vi "Test Camera + Joystick.vi"() -> ()   [LabVIEW 2019]
uses:
  Playground/Playground/Typedef/Barang.ctl
  Playground/Playground/Typedef/Kota.ctl
  <vilib>/vision/Instrument.llb/QR Code Search Options.ctl
  <vilib>/vision/Instrument.llb/Demodulation Mode.ctl
  <vilib>/vision/Instrument.llb/Cell Sample Size.ctl
  <vilib>/vision/Instrument.llb/Cell Filter Mode.ctl
  <vilib>/vision/Instrument.llb/QR Code Description Options.ctl
  <vilib>/vision/Instrument.llb/Data Matrix Polarity.ctl
  <vilib>/vision/Instrument.llb/QR Code Model Type.ctl
  <vilib>/userDefined/High Color/IMAQdx.ctl
  <vilib>/Utility/inputDevices.llb/joystickAcquire.vi
  <vilib>/Utility/inputDevices.llb/closeJoystick.vi
  <vilib>/vision/driver/NI_Vision_Acquisition_Software.lvlib
  <vilib>/vision/NI_Vision_Development_Module.lvlib
panel:
  out "axis info":T1
  out "error out":errorcluster
  in  "QR Description Options":T2={"Matrix Size (cells)"=0, "Barcode Polarity"=0, "Mirror Mode"=0, "QR Model"=3} {"Mirror Mode" items=["Auto-detect"=-2, "Normal"=0, "Mirrored"=1]; "Matrix Size (cells)" items=["Auto-detect"=0, "11x11 - Version 1 (Micro QR Only)"=11, "13x13 - Version 2 (Micro QR Only)"=13, "15x15 - Version 3 (Micro QR Only)"=15, "17x17 - Version 4 (Micro QR Only)"=17, "21x21 - Version 1"=21, "25x25 - Version 2"=25, "29x29 - Version 3"=29, "33x33 - Version 4"=33, "37x37 - Version 5"=37, "41x41 - Version 6"=41, "45x45 - Version 7"=45, "49x49 - Version 8"=49, "53x53 - Version 9"=53, "57x57 - Version 10"=57, "61x61 - Version 11"=61, "65x65 - Version 12"=65, "69x69 - Version 13"=69, "73x73 - Version 14"=73, "77x77 - Version 15"=77, "81x81 - Version 16"=81, "85x85 - Version 17"=85, "89x89 - Version 18"=89, "93x93 - Version 19"=93, "97x97 - Version 20"=97, "101x101 - Version 21"=101, "105x105 - Version 22"=105, "109x109 - Version 23"=109, "113x113 - Version 24"=113, "117x117 - Version 25"=117, "121x121 - Version 26"=121, "125x125 - Version 27"=125, "129x129 - Version 28"=129, "133x133 - Version 29"=133, "137x137 - Version 30"=137, "141x141 - Version 31"=141, "145x145 - Version 32"=145, "149x149 - Version 33"=149, "153x153 - Version 34"=153, "157x157 - Version 35"=157, "161x161 - Version 36"=161, "165x165 - Version 37"=165, "169x169 -  Version 38"=169, "173x173 - Version 39"=173, "177x177 - Version 40"=177]; "QR Model" items=["Auto-detect", "Micro", "Model 1", "Model 2"]; "Barcode Polarity" items=["Auto-detect"=-2, "Black on White"=0, "White on Black"=1]}
  in  "QR Code Cell Size (pixels)":cluster{"Minimum Size":u32, "Maximum Size":u32}={"Minimum Size"=3, "Maximum Size"=7}
  in  "QR Search Options":T5={"Rotation Mode"=enum."Unlimited", "Skip Location?"=FALSE, "Edge Threshold"=30, "Demodulation Mode"=0, "Cell Sample Size"=3, "Cell Filter Mode"=-2, "Skew Degrees Allowed"=5} {"Cell Filter Mode" items=["Auto-detect"=-2, "Average"=0, "Median"=1, "Central Average"=2, "High Average"=3, "Low Average"=4, "Very High Average"=5, "Very Low Average"=6, "All Filters"=8]; "Cell Sample Size" items=["Auto-detect"=-2, "1x1"=1, "2x2"=2, "3x3"=3, "4x4"=4, "5x5"=5, "6x6"=6, "7x7"=7]; "Demodulation Mode" items=["Auto-detect"=-2, "Histogram"=0, "Local Contrast"=1, "Combination"=2, "All"=3]}
  out "appended array":cluster{"Kota":T9, T10[], bool[]}[](array[cluster])
  out "output cluster":cluster{"Kota":T9, T10[], bool[]}
  out "Saved":bool
  out "Data num":dbl
  out "Image":T11(plugin-control)
  out "Found?":bool
  out "Data":string
  out "ROI":T11(plugin-control)
  in  "HSV Sample":T12(array[cluster])=[{"Red or Hue Range"={"Lower value"=240, "Upper value"=253}, "Green or Sat Range"={"Lower value"=4, "Upper value"=35}, "Blue or Luma or Val or Inten Range"={"Lower value"=115, "Upper value"=160}}, {"Red or Hue Range"={"Lower value"=102, "Upper value"=140}, "Green or Sat Range"={"Lower value"=6, "Upper value"=26}, "Blue or Luma or Val or Inten Range"={"Lower value"=112, "Upper value"=142}}, {"Red or Hue Range"={"Lower value"=149, "Upper value"=166}, "Green or Sat Range"={"Lower value"=6, "Upper value"=28}, "Blue or Luma or Val or Inten Range"={"Lower value"=106, "Upper value"=132}}, {"Red or Hue Range"={"Lower value"=146, "Upper value"=166}, "Green or Sat Range"={"Lower value"=7, "Upper value"=29}, "Blue or Luma or Val or Inten Range"={"Lower value"=108, "Upper value"=131}}, {"Red or Hue Range"={"Lower value"=146, "Upper value"=170}, "Green or Sat Range"={"Lower value"=7, "Upper value"=28}, "Blue or Luma or Val or Inten Range"={"Lower value"=106, "Upper value"=130}}, {"Red or Hue Range"={"Lower value"=146, "Upper value"=165}, "Green or Sat Range"={"Lower value"=6, "Upper value"=27}, "Blue or Luma or Val or Inten Range"={"Lower value"=106, "Upper value"=132}}, {"Red or Hue Range"={"Lower value"=145, "Upper value"=166}, "Green or Sat Range"={"Lower value"=6, "Upper value"=28}, "Blue or Luma or Val or Inten Range"={"Lower value"=108, "Upper value"=131}}, {"Red or Hue Range"={"Lower value"=146, "Upper value"=168}, "Green or Sat Range"={"Lower value"=7, "Upper value"=31}, "Blue or Luma or Val or Inten Range"={"Lower value"=108, "Upper value"=129}}, {"Red or Hue Range"={"Lower value"=146, "Upper value"=170}, "Green or Sat Range"={"Lower value"=7, "Upper value"=28}, "Blue or Luma or Val or Inten Range"={"Lower value"=108, "Upper value"=130}}, {"Red or Hue Range"={"Lower value"=146, "Upper value"=178}, "Green or Sat Range"={"Lower value"=5, "Upper value"=36}, "Blue or Luma or Val or Inten Range"={"Lower value"=105, "Upper value"=134}}, {"Red or Hue Range"={"Lower value"=142, "Upper value"=178}, "Green or Sat Range"={"Lower value"=4, "Upper value"=32}, "Blue or Luma or Val or Inten Range"={"Lower value"=104, "Upper value"=133}}, {"Red or Hue Range"={"Lower value"=149, "Upper value"=166}, "Green or Sat Range"={"Lower value"=10, "Upper value"=37}, "Blue or Luma or Val or Inten Range"={"Lower value"=110, "Upper value"=137}}, {"Red or Hue Range"={"Lower value"=149, "Upper value"=170}, "Green or Sat Range"={"Lower value"=9, "Upper value"=39}, "Blue or Luma or Val or Inten Range"={"Lower value"=110, "Upper value"=139}}, {"Red or Hue Range"={"Lower value"=106, "Upper value"=137}, "Green or Sat Range"={"Lower value"=7, "Upper value"=25}, "Blue or Luma or Val or Inten Range"={"Lower value"=114, "Upper value"=147}}, {"Red or Hue Range"={"Lower value"=228, "Upper value"=253}, "Green or Sat Range"={"Lower value"=4, "Upper value"=37}, "Blue or Luma or Val or Inten Range"={"Lower value"=114, "Upper value"=164}}, {"Red or Hue Range"={"Lower value"=237, "Upper value"=253}, "Green or Sat Range"={"Lower value"=6, "Upper value"=36}, "Blue or Luma or Val or Inten Range"={"Lower value"=114, "Upper value"=159}}, {"Red or Hue Range"={"Lower value"=0, "Upper value"=253}, "Green or Sat Range"={"Lower value"=6, "Upper value"=37}, "Blue or Luma or Val or Inten Range"={"Lower value"=114, "Upper value"=161}}, {"Red or Hue Range"={"Lower value"=140, "Upper value"=253}, "Green or Sat Range"={"Lower value"=2, "Upper value"=43}, "Blue or Luma or Val or Inten Range"={"Lower value"=109, "Upper value"=186}}, {"Red or Hue Range"={"Lower value"=140, "Upper value"=253}, "Green or Sat Range"={"Lower value"=2, "Upper value"=44}, "Blue or Luma or Val or Inten Range"={"Lower value"=108, "Upper value"=193}}, {"Red or Hue Range"={"Lower value"=0, "Upper value"=253}, "Green or Sat Range"={"Lower value"=2, "Upper value"=41}, "Blue or Luma or Val or Inten Range"={"Lower value"=108, "Upper value"=188}}, {"Red or Hue Range"={"Lower value"=0, "Upper value"=253}, "Green or Sat Range"={"Lower value"=2, "Upper value"=41}, "Blue or Luma or Val or Inten Range"={"Lower value"=109, "Upper value"=187}}, {"Red or Hue Range"={"Lower value"=239, "Upper value"=252}, "Green or Sat Range"={"Lower value"=14, "Upper value"=36}, "Blue or Luma or Val or Inten Range"={"Lower value"=132, "Upper value"=160}}, {"Red or Hue Range"={"Lower value"=110, "Upper value"=132}, "Green or Sat Range"={"Lower value"=7, "Upper value"=21}, "Blue or Luma or Val or Inten Range"={"Lower value"=115, "Upper value"=130}}, {"Red or Hue Range"={"Lower value"=145, "Upper value"=170}, "Green or Sat Range"={"Lower value"=10, "Upper value"=29}, "Blue or Luma or Val or Inten Range"={"Lower value"=112, "Upper value"=128}}, {"Red or Hue Range"={"Lower value"=147, "Upper value"=170}, "Green or Sat Range"={"Lower value"=8, "Upper value"=27}, "Blue or Luma or Val or Inten Range"={"Lower value"=111, "Upper value"=127}}, {"Red or Hue Range"={"Lower value"=150, "Upper value"=170}, "Green or Sat Range"={"Lower value"=10, "Upper value"=27}, "Blue or Luma or Val or Inten Range"={"Lower value"=113, "Upper value"=126}}, {"Red or Hue Range"={"Lower value"=149, "Upper value"=170}, "Green or Sat Range"={"Lower value"=8, "Upper value"=29}, "Blue or Luma or Val or Inten Range"={"Lower value"=112, "Upper value"=126}}, {"Red or Hue Range"={"Lower value"=109, "Upper value"=131}, "Green or Sat Range"={"Lower value"=7, "Upper value"=21}, "Blue or Luma or Val or Inten Range"={"Lower value"=115, "Upper value"=131}}, {"Red or Hue Range"={"Lower value"=109, "Upper value"=132}, "Green or Sat Range"={"Lower value"=7, "Upper value"=21}, "Blue or Luma or Val or Inten Range"={"Lower value"=115, "Upper value"=130}}, {"Red or Hue Range"={"Lower value"=109, "Upper value"=131}, "Green or Sat Range"={"Lower value"=8, "Upper value"=21}, "Blue or Luma or Val or Inten Range"={"Lower value"=115, "Upper value"=130}}, {"Red or Hue Range"={"Lower value"=239, "Upper value"=253}, "Green or Sat Range"={"Lower value"=15, "Upper value"=37}, "Blue or Luma or Val or Inten Range"={"Lower value"=129, "Upper value"=163}}, {"Red or Hue Range"={"Lower value"=239, "Upper value"=251}, "Green or Sat Range"={"Lower value"=15, "Upper value"=38}, "Blue or Luma or Val or Inten Range"={"Lower value"=128, "Upper value"=163}}, {"Red or Hue Range"={"Lower value"=239, "Upper value"=252}, "Green or Sat Range"={"Lower value"=15, "Upper value"=37}, "Blue or Luma or Val or Inten Range"={"Lower value"=128, "Upper value"=164}}, {"Red or Hue Range"={"Lower value"=240, "Upper value"=252}, "Green or Sat Range"={"Lower value"=17, "Upper value"=37}, "Blue or Luma or Val or Inten Range"={"Lower value"=132, "Upper value"=163}}, {"Red or Hue Range"={"Lower value"=239, "Upper value"=251}, "Green or Sat Range"={"Lower value"=16, "Upper value"=38}, "Blue or Luma or Val or Inten Range"={"Lower value"=132, "Upper value"=164}}, {"Red or Hue Range"={"Lower value"=239, "Upper value"=253}, "Green or Sat Range"={"Lower value"=16, "Upper value"=37}, "Blue or Luma or Val or Inten Range"={"Lower value"=134, "Upper value"=165}}, {"Red or Hue Range"={"Lower value"=245, "Upper value"=251}, "Green or Sat Range"={"Lower value"=59, "Upper value"=85}, "Blue or Luma or Val or Inten Range"={"Lower value"=171, "Upper value"=194}}, {"Red or Hue Range"={"Lower value"=112, "Upper value"=124}, "Green or Sat Range"={"Lower value"=23, "Upper value"=37}, "Blue or Luma or Val or Inten Range"={"Lower value"=121, "Upper value"=145}}, {"Red or Hue Range"={"Lower value"=112, "Upper value"=126}, "Green or Sat Range"={"Lower value"=23, "Upper value"=37}, "Blue or Luma or Val or Inten Range"={"Lower value"=121, "Upper value"=143}}, {"Red or Hue Range"={"Lower value"=112, "Upper value"=126}, "Green or Sat Range"={"Lower value"=23, "Upper value"=39}, "Blue or Luma or Val or Inten Range"={"Lower value"=119, "Upper value"=144}}, {"Red or Hue Range"={"Lower value"=112, "Upper value"=126}, "Green or Sat Range"={"Lower value"=24, "Upper value"=37}, "Blue or Luma or Val or Inten Range"={"Lower value"=118, "Upper value"=144}}, {"Red or Hue Range"={"Lower value"=245, "Upper value"=251}, "Green or Sat Range"={"Lower value"=63, "Upper value"=83}, "Blue or Luma or Val or Inten Range"={"Lower value"=173, "Upper value"=192}}, {"Red or Hue Range"={"Lower value"=245, "Upper value"=251}, "Green or Sat Range"={"Lower value"=60, "Upper value"=85}, "Blue or Luma or Val or Inten Range"={"Lower value"=172, "Upper value"=194}}, {"Red or Hue Range"={"Lower value"=245, "Upper value"=251}, "Green or Sat Range"={"Lower value"=57, "Upper value"=81}, "Blue or Luma or Val or Inten Range"={"Lower value"=169, "Upper value"=191}}, {"Red or Hue Range"={"Lower value"=245, "Upper value"=251}, "Green or Sat Range"={"Lower value"=57, "Upper value"=88}, "Blue or Luma or Val or Inten Range"={"Lower value"=169, "Upper value"=195}}, {"Red or Hue Range"={"Lower value"=245, "Upper value"=251}, "Green or Sat Range"={"Lower value"=56, "Upper value"=83}, "Blue or Luma or Val or Inten Range"={"Lower value"=169, "Upper value"=192}}, {"Red or Hue Range"={"Lower value"=245, "Upper value"=251}, "Green or Sat Range"={"Lower value"=60, "Upper value"=87}, "Blue or Luma or Val or Inten Range"={"Lower value"=171, "Upper value"=193}}, {"Red or Hue Range"={"Lower value"=245, "Upper value"=250}, "Green or Sat Range"={"Lower value"=59, "Upper value"=86}, "Blue or Luma or Val or Inten Range"={"Lower value"=172, "Upper value"=194}}, {"Red or Hue Range"={"Lower value"=246, "Upper value"=251}, "Green or Sat Range"={"Lower value"=60, "Upper value"=87}, "Blue or Luma or Val or Inten Range"={"Lower value"=171, "Upper value"=194}}, {"Red or Hue Range"={"Lower value"=244, "Upper value"=251}, "Green or Sat Range"={"Lower value"=61, "Upper value"=87}, "Blue or Luma or Val or Inten Range"={"Lower value"=171, "Upper value"=194}}, {"Red or Hue Range"={"Lower value"=244, "Upper value"=251}, "Green or Sat Range"={"Lower value"=60, "Upper value"=87}, "Blue or Luma or Val or Inten Range"={"Lower value"=170, "Upper value"=194}}, {"Red or Hue Range"={"Lower value"=246, "Upper value"=251}, "Green or Sat Range"={"Lower value"=63, "Upper value"=86}, "Blue or Luma or Val or Inten Range"={"Lower value"=173, "Upper value"=193}}, {"Red or Hue Range"={"Lower value"=246, "Upper value"=250}, "Green or Sat Range"={"Lower value"=60, "Upper value"=87}, "Blue or Luma or Val or Inten Range"={"Lower value"=170, "Upper value"=194}}, {"Red or Hue Range"={"Lower value"=250, "Upper value"=255}, "Green or Sat Range"={"Lower value"=70, "Upper value"=125}, "Blue or Luma or Val or Inten Range"={"Lower value"=167, "Upper value"=207}}, {"Red or Hue Range"={"Lower value"=0, "Upper value"=255}, "Green or Sat Range"={"Lower value"=65, "Upper value"=121}, "Blue or Luma or Val or Inten Range"={"Lower value"=162, "Upper value"=206}}, {"Red or Hue Range"={"Lower value"=0, "Upper value"=255}, "Green or Sat Range"={"Lower value"=52, "Upper value"=164}, "Blue or Luma or Val or Inten Range"={"Lower value"=152, "Upper value"=228}}, {"Red or Hue Range"={"Lower value"=0, "Upper value"=255}, "Green or Sat Range"={"Lower value"=51, "Upper value"=166}, "Blue or Luma or Val or Inten Range"={"Lower value"=153, "Upper value"=228}}, {"Red or Hue Range"={"Lower value"=0, "Upper value"=255}, "Green or Sat Range"={"Lower value"=51, "Upper value"=172}, "Blue or Luma or Val or Inten Range"={"Lower value"=149, "Upper value"=231}}, {"Red or Hue Range"={"Lower value"=251, "Upper value"=254}, "Green or Sat Range"={"Lower value"=62, "Upper value"=110}, "Blue or Luma or Val or Inten Range"={"Lower value"=160, "Upper value"=195}}, {"Red or Hue Range"={"Lower value"=0, "Upper value"=254}, "Green or Sat Range"={"Lower value"=65, "Upper value"=110}, "Blue or Luma or Val or Inten Range"={"Lower value"=162, "Upper value"=196}}, {"Red or Hue Range"={"Lower value"=0, "Upper value"=254}, "Green or Sat Range"={"Lower value"=63, "Upper value"=109}, "Blue or Luma or Val or Inten Range"={"Lower value"=160, "Upper value"=195}}, {"Red or Hue Range"={"Lower value"=250, "Upper value"=255}, "Green or Sat Range"={"Lower value"=87, "Upper value"=125}, "Blue or Luma or Val or Inten Range"={"Lower value"=182, "Upper value"=207}}, {"Red or Hue Range"={"Lower value"=0, "Upper value"=255}, "Green or Sat Range"={"Lower value"=84, "Upper value"=127}, "Blue or Luma or Val or Inten Range"={"Lower value"=181, "Upper value"=209}}, {"Red or Hue Range"={"Lower value"=0, "Upper value"=255}, "Green or Sat Range"={"Lower value"=83, "Upper value"=125}, "Blue or Luma or Val or Inten Range"={"Lower value"=180, "Upper value"=207}}, {"Red or Hue Range"={"Lower value"=0, "Upper value"=255}, "Green or Sat Range"={"Lower value"=66, "Upper value"=144}, "Blue or Luma or Val or Inten Range"={"Lower value"=167, "Upper value"=214}}, {"Red or Hue Range"={"Lower value"=104, "Upper value"=114}, "Green or Sat Range"={"Lower value"=58, "Upper value"=113}, "Blue or Luma or Val or Inten Range"={"Lower value"=146, "Upper value"=199}}, {"Red or Hue Range"={"Lower value"=105, "Upper value"=115}, "Green or Sat Range"={"Lower value"=57, "Upper value"=114}, "Blue or Luma or Val or Inten Range"={"Lower value"=143, "Upper value"=200}}, {"Red or Hue Range"={"Lower value"=103, "Upper value"=115}, "Green or Sat Range"={"Lower value"=58, "Upper value"=111}, "Blue or Luma or Val or Inten Range"={"Lower value"=142, "Upper value"=196}}, {"Red or Hue Range"={"Lower value"=0, "Upper value"=255}, "Green or Sat Range"={"Lower value"=0, "Upper value"=255}, "Blue or Luma or Val or Inten Range"={"Lower value"=98, "Upper value"=255}}, {"Red or Hue Range"={"Lower value"=0, "Upper value"=255}, "Green or Sat Range"={"Lower value"=0, "Upper value"=255}, "Blue or Luma or Val or Inten Range"={"Lower value"=98, "Upper value"=255}}, {"Red or Hue Range"={"Lower value"=0, "Upper value"=255}, "Green or Sat Range"={"Lower value"=0, "Upper value"=255}, "Blue or Luma or Val or Inten Range"={"Lower value"=96, "Upper value"=255}}, {"Red or Hue Range"={"Lower value"=105, "Upper value"=114}, "Green or Sat Range"={"Lower value"=70, "Upper value"=120}, "Blue or Luma or Val or Inten Range"={"Lower value"=162, "Upper value"=199}}, {"Red or Hue Range"={"Lower value"=105, "Upper value"=113}, "Green or Sat Range"={"Lower value"=70, "Upper value"=116}, "Blue or Luma or Val or Inten Range"={"Lower value"=162, "Upper value"=199}}, {"Red or Hue Range"={"Lower value"=106, "Upper value"=114}, "Green or Sat Range"={"Lower value"=48, "Upper value"=68}, "Blue or Luma or Val or Inten Range"={"Lower value"=143, "Upper value"=164}}, {"Red or Hue Range"={"Lower value"=103, "Upper value"=114}, "Green or Sat Range"={"Lower value"=51, "Upper value"=68}, "Blue or Luma or Val or Inten Range"={"Lower value"=143, "Upper value"=162}}, {"Red or Hue Range"={"Lower value"=105, "Upper value"=117}, "Green or Sat Range"={"Lower value"=48, "Upper value"=70}, "Blue or Luma or Val or Inten Range"={"Lower value"=142, "Upper value"=161}}, {"Red or Hue Range"={"Lower value"=247, "Upper value"=255}, "Green or Sat Range"={"Lower value"=64, "Upper value"=148}, "Blue or Luma or Val or Inten Range"={"Lower value"=167, "Upper value"=216}}, {"Red or Hue Range"={"Lower value"=0, "Upper value"=255}, "Green or Sat Range"={"Lower value"=62, "Upper value"=145}, "Blue or Luma or Val or Inten Range"={"Lower value"=165, "Upper value"=215}}, {"Red or Hue Range"={"Lower value"=249, "Upper value"=255}, "Green or Sat Range"={"Lower value"=64, "Upper value"=142}, "Blue or Luma or Val or Inten Range"={"Lower value"=167, "Upper value"=213}}, {"Red or Hue Range"={"Lower value"=249, "Upper value"=255}, "Green or Sat Range"={"Lower value"=102, "Upper value"=143}, "Blue or Luma or Val or Inten Range"={"Lower value"=194, "Upper value"=213}}, {"Red or Hue Range"={"Lower value"=250, "Upper value"=255}, "Green or Sat Range"={"Lower value"=121, "Upper value"=146}, "Blue or Luma or Val or Inten Range"={"Lower value"=201, "Upper value"=216}}, {"Red or Hue Range"={"Lower value"=0, "Upper value"=255}, "Green or Sat Range"={"Lower value"=113, "Upper value"=255}, "Blue or Luma or Val or Inten Range"={"Lower value"=208, "Upper value"=255}}, {"Red or Hue Range"={"Lower value"=0, "Upper value"=255}, "Green or Sat Range"={"Lower value"=113, "Upper value"=255}, "Blue or Luma or Val or Inten Range"={"Lower value"=208, "Upper value"=255}}, {"Red or Hue Range"={"Lower value"=0, "Upper value"=255}, "Green or Sat Range"={"Lower value"=118, "Upper value"=255}, "Blue or Luma or Val or Inten Range"={"Lower value"=210, "Upper value"=255}}, {"Red or Hue Range"={"Lower value"=0, "Upper value"=255}, "Green or Sat Range"={"Lower value"=111, "Upper value"=255}, "Blue or Luma or Val or Inten Range"={"Lower value"=206, "Upper value"=255}}, {"Red or Hue Range"={"Lower value"=0, "Upper value"=255}, "Green or Sat Range"={"Lower value"=0, "Upper value"=255}, "Blue or Luma or Val or Inten Range"={"Lower value"=101, "Upper value"=255}}, {"Red or Hue Range"={"Lower value"=0, "Upper value"=255}, "Green or Sat Range"={"Lower value"=0, "Upper value"=255}, "Blue or Luma or Val or Inten Range"={"Lower value"=100, "Upper value"=255}}, {"Red or Hue Range"={"Lower value"=0, "Upper value"=255}, "Green or Sat Range"={"Lower value"=0, "Upper value"=255}, "Blue or Luma or Val or Inten Range"={"Lower value"=99, "Upper value"=255}}, {"Red or Hue Range"={"Lower value"=0, "Upper value"=255}, "Green or Sat Range"={"Lower value"=0, "Upper value"=255}, "Blue or Luma or Val or Inten Range"={"Lower value"=98, "Upper value"=255}}, {"Red or Hue Range"={"Lower value"=0, "Upper value"=255}, "Green or Sat Range"={"Lower value"=108, "Upper value"=188}, "Blue or Luma or Val or Inten Range"={"Lower value"=195, "Upper value"=234}}, {"Red or Hue Range"={"Lower value"=0, "Upper value"=255}, "Green or Sat Range"={"Lower value"=109, "Upper value"=190}, "Blue or Luma or Val or Inten Range"={"Lower value"=195, "Upper value"=234}}, {"Red or Hue Range"={"Lower value"=0, "Upper value"=255}, "Green or Sat Range"={"Lower value"=107, "Upper value"=196}, "Blue or Luma or Val or Inten Range"={"Lower value"=195, "Upper value"=236}}, {"Red or Hue Range"={"Lower value"=0, "Upper value"=255}, "Green or Sat Range"={"Lower value"=106, "Upper value"=195}, "Blue or Luma or Val or Inten Range"={"Lower value"=195, "Upper value"=235}}, {"Red or Hue Range"={"Lower value"=0, "Upper value"=255}, "Green or Sat Range"={"Lower value"=107, "Upper value"=189}, "Blue or Luma or Val or Inten Range"={"Lower value"=195, "Upper value"=234}}, {"Red or Hue Range"={"Lower value"=0, "Upper value"=255}, "Green or Sat Range"={"Lower value"=108, "Upper value"=190}, "Blue or Luma or Val or Inten Range"={"Lower value"=195, "Upper value"=234}}, {"Red or Hue Range"={"Lower value"=0, "Upper value"=255}, "Green or Sat Range"={"Lower value"=107, "Upper value"=194}, "Blue or Luma or Val or Inten Range"={"Lower value"=195, "Upper value"=235}}, {"Red or Hue Range"={"Lower value"=0, "Upper value"=255}, "Green or Sat Range"={"Lower value"=108, "Upper value"=190}, "Blue or Luma or Val or Inten Range"={"Lower value"=195, "Upper value"=234}}, {"Red or Hue Range"={"Lower value"=0, "Upper value"=255}, "Green or Sat Range"={"Lower value"=107, "Upper value"=188}, "Blue or Luma or Val or Inten Range"={"Lower value"=195, "Upper value"=234}}, {"Red or Hue Range"={"Lower value"=0, "Upper value"=255}, "Green or Sat Range"={"Lower value"=106, "Upper value"=190}, "Blue or Luma or Val or Inten Range"={"Lower value"=193, "Upper value"=234}}, {"Red or Hue Range"={"Lower value"=0, "Upper value"=255}, "Green or Sat Range"={"Lower value"=108, "Upper value"=190}, "Blue or Luma or Val or Inten Range"={"Lower value"=195, "Upper value"=234}}, {"Red or Hue Range"={"Lower value"=0, "Upper value"=255}, "Green or Sat Range"={"Lower value"=106, "Upper value"=194}, "Blue or Luma or Val or Inten Range"={"Lower value"=193, "Upper value"=235}}, {"Red or Hue Range"={"Lower value"=0, "Upper value"=255}, "Green or Sat Range"={"Lower value"=106, "Upper value"=190}, "Blue or Luma or Val or Inten Range"={"Lower value"=195, "Upper value"=234}}, {"Red or Hue Range"={"Lower value"=0, "Upper value"=255}, "Green or Sat Range"={"Lower value"=105, "Upper value"=187}, "Blue or Luma or Val or Inten Range"={"Lower value"=193, "Upper value"=233}}, {"Red or Hue Range"={"Lower value"=0, "Upper value"=255}, "Green or Sat Range"={"Lower value"=107, "Upper value"=189}, "Blue or Luma or Val or Inten Range"={"Lower value"=195, "Upper value"=234}}, {"Red or Hue Range"={"Lower value"=0, "Upper value"=255}, "Green or Sat Range"={"Lower value"=107, "Upper value"=190}, "Blue or Luma or Val or Inten Range"={"Lower value"=193, "Upper value"=234}}, {"Red or Hue Range"={"Lower value"=0, "Upper value"=255}, "Green or Sat Range"={"Lower value"=106, "Upper value"=185}, "Blue or Luma or Val or Inten Range"={"Lower value"=195, "Upper value"=232}}, {"Red or Hue Range"={"Lower value"=0, "Upper value"=255}, "Green or Sat Range"={"Lower value"=109, "Upper value"=186}, "Blue or Luma or Val or Inten Range"={"Lower value"=196, "Upper value"=232}}, {"Red or Hue Range"={"Lower value"=0, "Upper value"=255}, "Green or Sat Range"={"Lower value"=108, "Upper value"=187}, "Blue or Luma or Val or Inten Range"={"Lower value"=195, "Upper value"=232}}, {"Red or Hue Range"={"Lower value"=0, "Upper value"=255}, "Green or Sat Range"={"Lower value"=105, "Upper value"=184}, "Blue or Luma or Val or Inten Range"={"Lower value"=196, "Upper value"=232}}, {"Red or Hue Range"={"Lower value"=0, "Upper value"=255}, "Green or Sat Range"={"Lower value"=102, "Upper value"=189}, "Blue or Luma or Val or Inten Range"={"Lower value"=196, "Upper value"=233}}, {"Red or Hue Range"={"Lower value"=0, "Upper value"=255}, "Green or Sat Range"={"Lower value"=108, "Upper value"=185}, "Blue or Luma or Val or Inten Range"={"Lower value"=194, "Upper value"=232}}, {"Red or Hue Range"={"Lower value"=0, "Upper value"=255}, "Green or Sat Range"={"Lower value"=107, "Upper value"=186}, "Blue or Luma or Val or Inten Range"={"Lower value"=196, "Upper value"=232}}, {"Red or Hue Range"={"Lower value"=0, "Upper value"=255}, "Green or Sat Range"={"Lower value"=108, "Upper value"=186}, "Blue or Luma or Val or Inten Range"={"Lower value"=195, "Upper value"=232}}, {"Red or Hue Range"={"Lower value"=0, "Upper value"=255}, "Green or Sat Range"={"Lower value"=103, "Upper value"=186}, "Blue or Luma or Val or Inten Range"={"Lower value"=195, "Upper value"=232}}, {"Red or Hue Range"={"Lower value"=0, "Upper value"=255}, "Green or Sat Range"={"Lower value"=104, "Upper value"=186}, "Blue or Luma or Val or Inten Range"={"Lower value"=193, "Upper value"=232}}, {"Red or Hue Range"={"Lower value"=0, "Upper value"=255}, "Green or Sat Range"={"Lower value"=106, "Upper value"=186}, "Blue or Luma or Val or Inten Range"={"Lower value"=196, "Upper value"=232}}, {"Red or Hue Range"={"Lower value"=0, "Upper value"=255}, "Green or Sat Range"={"Lower value"=110, "Upper value"=186}, "Blue or Luma or Val or Inten Range"={"Lower value"=196, "Upper value"=232}}, {"Red or Hue Range"={"Lower value"=0, "Upper value"=255}, "Green or Sat Range"={"Lower value"=107, "Upper value"=184}, "Blue or Luma or Val or Inten Range"={"Lower value"=196, "Upper value"=232}}, {"Red or Hue Range"={"Lower value"=0, "Upper value"=255}, "Green or Sat Range"={"Lower value"=106, "Upper value"=191}, "Blue or Luma or Val or Inten Range"={"Lower value"=196, "Upper value"=234}}, {"Red or Hue Range"={"Lower value"=0, "Upper value"=255}, "Green or Sat Range"={"Lower value"=111, "Upper value"=190}, "Blue or Luma or Val or Inten Range"={"Lower value"=196, "Upper value"=234}}, {"Red or Hue Range"={"Lower value"=0, "Upper value"=255}, "Green or Sat Range"={"Lower value"=107, "Upper value"=185}, "Blue or Luma or Val or Inten Range"={"Lower value"=197, "Upper value"=232}}, {"Red or Hue Range"={"Lower value"=0, "Upper value"=255}, "Green or Sat Range"={"Lower value"=83, "Upper value"=118}, "Blue or Luma or Val or Inten Range"={"Lower value"=175, "Upper value"=198}}, {"Red or Hue Range"={"Lower value"=78, "Upper value"=100}, "Green or Sat Range"={"Lower value"=15, "Upper value"=36}, "Blue or Luma or Val or Inten Range"={"Lower value"=81, "Upper value"=101}}, {"Red or Hue Range"={"Lower value"=83, "Upper value"=97}, "Green or Sat Range"={"Lower value"=15, "Upper value"=37}, "Blue or Luma or Val or Inten Range"={"Lower value"=83, "Upper value"=99}}, {"Red or Hue Range"={"Lower value"=80, "Upper value"=99}, "Green or Sat Range"={"Lower value"=15, "Upper value"=36}, "Blue or Luma or Val or Inten Range"={"Lower value"=81, "Upper value"=100}}, {"Red or Hue Range"={"Lower value"=80, "Upper value"=97}, "Green or Sat Range"={"Lower value"=14, "Upper value"=36}, "Blue or Luma or Val or Inten Range"={"Lower value"=81, "Upper value"=97}}, {"Red or Hue Range"={"Lower value"=83, "Upper value"=100}, "Green or Sat Range"={"Lower value"=15, "Upper value"=37}, "Blue or Luma or Val or Inten Range"={"Lower value"=83, "Upper value"=100}}, {"Red or Hue Range"={"Lower value"=81, "Upper value"=99}, "Green or Sat Range"={"Lower value"=15, "Upper value"=34}, "Blue or Luma or Val or Inten Range"={"Lower value"=82, "Upper value"=101}}, {"Red or Hue Range"={"Lower value"=83, "Upper value"=98}, "Green or Sat Range"={"Lower value"=12, "Upper value"=36}, "Blue or Luma or Val or Inten Range"={"Lower value"=81, "Upper value"=101}}, {"Red or Hue Range"={"Lower value"=83, "Upper value"=99}, "Green or Sat Range"={"Lower value"=15, "Upper value"=41}, "Blue or Luma or Val or Inten Range"={"Lower value"=82, "Upper value"=100}}, {"Red or Hue Range"={"Lower value"=81, "Upper value"=97}, "Green or Sat Range"={"Lower value"=15, "Upper value"=37}, "Blue or Luma or Val or Inten Range"={"Lower value"=81, "Upper value"=100}}, {"Red or Hue Range"={"Lower value"=78, "Upper value"=96}, "Green or Sat Range"={"Lower value"=15, "Upper value"=37}, "Blue or Luma or Val or Inten Range"={"Lower value"=81, "Upper value"=101}}, {"Red or Hue Range"={"Lower value"=0, "Upper value"=255}, "Green or Sat Range"={"Lower value"=81, "Upper value"=119}, "Blue or Luma or Val or Inten Range"={"Lower value"=173, "Upper value"=200}}, {"Red or Hue Range"={"Lower value"=0, "Upper value"=255}, "Green or Sat Range"={"Lower value"=81, "Upper value"=118}, "Blue or Luma or Val or Inten Range"={"Lower value"=175, "Upper value"=198}}, {"Red or Hue Range"={"Lower value"=0, "Upper value"=255}, "Green or Sat Range"={"Lower value"=81, "Upper value"=119}, "Blue or Luma or Val or Inten Range"={"Lower value"=174, "Upper value"=201}}, {"Red or Hue Range"={"Lower value"=0, "Upper value"=255}, "Green or Sat Range"={"Lower value"=83, "Upper value"=123}, "Blue or Luma or Val or Inten Range"={"Lower value"=177, "Upper value"=201}}, {"Red or Hue Range"={"Lower value"=0, "Upper value"=255}, "Green or Sat Range"={"Lower value"=79, "Upper value"=118}, "Blue or Luma or Val or Inten Range"={"Lower value"=173, "Upper value"=198}}, {"Red or Hue Range"={"Lower value"=0, "Upper value"=255}, "Green or Sat Range"={"Lower value"=79, "Upper value"=118}, "Blue or Luma or Val or Inten Range"={"Lower value"=173, "Upper value"=199}}, {"Red or Hue Range"={"Lower value"=0, "Upper value"=255}, "Green or Sat Range"={"Lower value"=75, "Upper value"=120}, "Blue or Luma or Val or Inten Range"={"Lower value"=171, "Upper value"=199}}, {"Red or Hue Range"={"Lower value"=0, "Upper value"=255}, "Green or Sat Range"={"Lower value"=84, "Upper value"=117}, "Blue or Luma or Val or Inten Range"={"Lower value"=175, "Upper value"=200}}, {"Red or Hue Range"={"Lower value"=0, "Upper value"=255}, "Green or Sat Range"={"Lower value"=82, "Upper value"=121}, "Blue or Luma or Val or Inten Range"={"Lower value"=172, "Upper value"=199}}, {"Red or Hue Range"={"Lower value"=0, "Upper value"=255}, "Green or Sat Range"={"Lower value"=10, "Upper value"=151}, "Blue or Luma or Val or Inten Range"={"Lower value"=160, "Upper value"=223}}, {"Red or Hue Range"={"Lower value"=0, "Upper value"=255}, "Green or Sat Range"={"Lower value"=16, "Upper value"=165}, "Blue or Luma or Val or Inten Range"={"Lower value"=155, "Upper value"=229}}, {"Red or Hue Range"={"Lower value"=0, "Upper value"=255}, "Green or Sat Range"={"Lower value"=25, "Upper value"=160}, "Blue or Luma or Val or Inten Range"={"Lower value"=152, "Upper value"=229}}, {"Red or Hue Range"={"Lower value"=0, "Upper value"=255}, "Green or Sat Range"={"Lower value"=10, "Upper value"=154}, "Blue or Luma or Val or Inten Range"={"Lower value"=157, "Upper value"=224}}, {"Red or Hue Range"={"Lower value"=0, "Upper value"=255}, "Green or Sat Range"={"Lower value"=22, "Upper value"=158}, "Blue or Luma or Val or Inten Range"={"Lower value"=155, "Upper value"=226}}, {"Red or Hue Range"={"Lower value"=0, "Upper value"=255}, "Green or Sat Range"={"Lower value"=26, "Upper value"=148}, "Blue or Luma or Val or Inten Range"={"Lower value"=151, "Upper value"=221}}, {"Red or Hue Range"={"Lower value"=0, "Upper value"=255}, "Green or Sat Range"={"Lower value"=14, "Upper value"=150}, "Blue or Luma or Val or Inten Range"={"Lower value"=161, "Upper value"=222}}, {"Red or Hue Range"={"Lower value"=0, "Upper value"=254}, "Green or Sat Range"={"Lower value"=46, "Upper value"=86}, "Blue or Luma or Val or Inten Range"={"Lower value"=102, "Upper value"=159}}, {"Red or Hue Range"={"Lower value"=0, "Upper value"=254}, "Green or Sat Range"={"Lower value"=45, "Upper value"=86}, "Blue or Luma or Val or Inten Range"={"Lower value"=98, "Upper value"=156}}, {"Red or Hue Range"={"Lower value"=0, "Upper value"=254}, "Green or Sat Range"={"Lower value"=35, "Upper value"=86}, "Blue or Luma or Val or Inten Range"={"Lower value"=92, "Upper value"=158}}, {"Red or Hue Range"={"Lower value"=0, "Upper value"=254}, "Green or Sat Range"={"Lower value"=45, "Upper value"=89}, "Blue or Luma or Val or Inten Range"={"Lower value"=100, "Upper value"=163}}, {"Red or Hue Range"={"Lower value"=0, "Upper value"=254}, "Green or Sat Range"={"Lower value"=42, "Upper value"=85}, "Blue or Luma or Val or Inten Range"={"Lower value"=100, "Upper value"=163}}, {"Red or Hue Range"={"Lower value"=0, "Upper value"=254}, "Green or Sat Range"={"Lower value"=46, "Upper value"=87}, "Blue or Luma or Val or Inten Range"={"Lower value"=102, "Upper value"=162}}, {"Red or Hue Range"={"Lower value"=0, "Upper value"=254}, "Green or Sat Range"={"Lower value"=47, "Upper value"=88}, "Blue or Luma or Val or Inten Range"={"Lower value"=102, "Upper value"=153}}, {"Red or Hue Range"={"Lower value"=0, "Upper value"=254}, "Green or Sat Range"={"Lower value"=46, "Upper value"=89}, "Blue or Luma or Val or Inten Range"={"Lower value"=101, "Upper value"=155}}, {"Red or Hue Range"={"Lower value"=0, "Upper value"=254}, "Green or Sat Range"={"Lower value"=41, "Upper value"=86}, "Blue or Luma or Val or Inten Range"={"Lower value"=98, "Upper value"=162}}, {"Red or Hue Range"={"Lower value"=0, "Upper value"=254}, "Green or Sat Range"={"Lower value"=46, "Upper value"=85}, "Blue or Luma or Val or Inten Range"={"Lower value"=102, "Upper value"=159}}, {"Red or Hue Range"={"Lower value"=0, "Upper value"=254}, "Green or Sat Range"={"Lower value"=47, "Upper value"=89}, "Blue or Luma or Val or Inten Range"={"Lower value"=99, "Upper value"=157}}, {"Red or Hue Range"={"Lower value"=0, "Upper value"=254}, "Green or Sat Range"={"Lower value"=42, "Upper value"=87}, "Blue or Luma or Val or Inten Range"={"Lower value"=95, "Upper value"=160}}, {"Red or Hue Range"={"Lower value"=0, "Upper value"=254}, "Green or Sat Range"={"Lower value"=46, "Upper value"=89}, "Blue or Luma or Val or Inten Range"={"Lower value"=102, "Upper value"=157}}, {"Red or Hue Range"={"Lower value"=0, "Upper value"=254}, "Green or Sat Range"={"Lower value"=43, "Upper value"=87}, "Blue or Luma or Val or Inten Range"={"Lower value"=100, "Upper value"=158}}, {"Red or Hue Range"={"Lower value"=0, "Upper value"=254}, "Green or Sat Range"={"Lower value"=41, "Upper value"=85}, "Blue or Luma or Val or Inten Range"={"Lower value"=96, "Upper value"=160}}, {"Red or Hue Range"={"Lower value"=0, "Upper value"=254}, "Green or Sat Range"={"Lower value"=37, "Upper value"=87}, "Blue or Luma or Val or Inten Range"={"Lower value"=95, "Upper value"=160}}, {"Red or Hue Range"={"Lower value"=0, "Upper value"=254}, "Green or Sat Range"={"Lower value"=41, "Upper value"=86}, "Blue or Luma or Val or Inten Range"={"Lower value"=98, "Upper value"=158}}, {"Red or Hue Range"={"Lower value"=0, "Upper value"=255}, "Green or Sat Range"={"Lower value"=51, "Upper value"=210}, "Blue or Luma or Val or Inten Range"={"Lower value"=162, "Upper value"=241}}, {"Red or Hue Range"={"Lower value"=86, "Upper value"=121}, "Green or Sat Range"={"Lower value"=45, "Upper value"=137}, "Blue or Luma or Val or Inten Range"={"Lower value"=151, "Upper value"=201}}, {"Red or Hue Range"={"Lower value"=85, "Upper value"=120}, "Green or Sat Range"={"Lower value"=55, "Upper value"=135}, "Blue or Luma or Val or Inten Range"={"Lower value"=154, "Upper value"=200}}, {"Red or Hue Range"={"Lower value"=85, "Upper value"=120}, "Green or Sat Range"={"Lower value"=57, "Upper value"=135}, "Blue or Luma or Val or Inten Range"={"Lower value"=153, "Upper value"=199}}, {"Red or Hue Range"={"Lower value"=85, "Upper value"=122}, "Green or Sat Range"={"Lower value"=45, "Upper value"=136}, "Blue or Luma or Val or Inten Range"={"Lower value"=150, "Upper value"=201}}, {"Red or Hue Range"={"Lower value"=85, "Upper value"=121}, "Green or Sat Range"={"Lower value"=57, "Upper value"=137}, "Blue or Luma or Val or Inten Range"={"Lower value"=151, "Upper value"=200}}, {"Red or Hue Range"={"Lower value"=83, "Upper value"=120}, "Green or Sat Range"={"Lower value"=45, "Upper value"=134}, "Blue or Luma or Val or Inten Range"={"Lower value"=150, "Upper value"=204}}, {"Red or Hue Range"={"Lower value"=86, "Upper value"=119}, "Green or Sat Range"={"Lower value"=51, "Upper value"=138}, "Blue or Luma or Val or Inten Range"={"Lower value"=152, "Upper value"=201}}, {"Red or Hue Range"={"Lower value"=85, "Upper value"=121}, "Green or Sat Range"={"Lower value"=45, "Upper value"=136}, "Blue or Luma or Val or Inten Range"={"Lower value"=151, "Upper value"=202}}, {"Red or Hue Range"={"Lower value"=84, "Upper value"=118}, "Green or Sat Range"={"Lower value"=35, "Upper value"=136}, "Blue or Luma or Val or Inten Range"={"Lower value"=148, "Upper value"=204}}, {"Red or Hue Range"={"Lower value"=85, "Upper value"=121}, "Green or Sat Range"={"Lower value"=45, "Upper value"=136}, "Blue or Luma or Val or Inten Range"={"Lower value"=151, "Upper value"=200}}, {"Red or Hue Range"={"Lower value"=82, "Upper value"=126}, "Green or Sat Range"={"Lower value"=21, "Upper value"=155}, "Blue or Luma or Val or Inten Range"={"Lower value"=142, "Upper value"=230}}, {"Red or Hue Range"={"Lower value"=85, "Upper value"=127}, "Green or Sat Range"={"Lower value"=21, "Upper value"=151}, "Blue or Luma or Val or Inten Range"={"Lower value"=144, "Upper value"=228}}, {"Red or Hue Range"={"Lower value"=81, "Upper value"=127}, "Green or Sat Range"={"Lower value"=17, "Upper value"=145}, "Blue or Luma or Val or Inten Range"={"Lower value"=142, "Upper value"=227}}, {"Red or Hue Range"={"Lower value"=85, "Upper value"=127}, "Green or Sat Range"={"Lower value"=25, "Upper value"=142}, "Blue or Luma or Val or Inten Range"={"Lower value"=147, "Upper value"=226}}, {"Red or Hue Range"={"Lower value"=80, "Upper value"=129}, "Green or Sat Range"={"Lower value"=23, "Upper value"=151}, "Blue or Luma or Val or Inten Range"={"Lower value"=147, "Upper value"=229}}, {"Red or Hue Range"={"Lower value"=75, "Upper value"=126}, "Green or Sat Range"={"Lower value"=23, "Upper value"=152}, "Blue or Luma or Val or Inten Range"={"Lower value"=144, "Upper value"=228}}, {"Red or Hue Range"={"Lower value"=85, "Upper value"=127}, "Green or Sat Range"={"Lower value"=21, "Upper value"=145}, "Blue or Luma or Val or Inten Range"={"Lower value"=139, "Upper value"=226}}, {"Red or Hue Range"={"Lower value"=85, "Upper value"=127}, "Green or Sat Range"={"Lower value"=20, "Upper value"=147}, "Blue or Luma or Val or Inten Range"={"Lower value"=149, "Upper value"=229}}, {"Red or Hue Range"={"Lower value"=85, "Upper value"=127}, "Green or Sat Range"={"Lower value"=21, "Upper value"=151}, "Blue or Luma or Val or Inten Range"={"Lower value"=144, "Upper value"=227}}, {"Red or Hue Range"={"Lower value"=85, "Upper value"=127}, "Green or Sat Range"={"Lower value"=22, "Upper value"=149}, "Blue or Luma or Val or Inten Range"={"Lower value"=145, "Upper value"=226}}, {"Red or Hue Range"={"Lower value"=85, "Upper value"=129}, "Green or Sat Range"={"Lower value"=21, "Upper value"=141}, "Blue or Luma or Val or Inten Range"={"Lower value"=146, "Upper value"=227}}, {"Red or Hue Range"={"Lower value"=85, "Upper value"=127}, "Green or Sat Range"={"Lower value"=23, "Upper value"=146}, "Blue or Luma or Val or Inten Range"={"Lower value"=148, "Upper value"=228}}, {"Red or Hue Range"={"Lower value"=83, "Upper value"=130}, "Green or Sat Range"={"Lower value"=29, "Upper value"=150}, "Blue or Luma or Val or Inten Range"={"Lower value"=146, "Upper value"=227}}, {"Red or Hue Range"={"Lower value"=85, "Upper value"=127}, "Green or Sat Range"={"Lower value"=23, "Upper value"=142}, "Blue or Luma or Val or Inten Range"={"Lower value"=145, "Upper value"=226}}, {"Red or Hue Range"={"Lower value"=83, "Upper value"=128}, "Green or Sat Range"={"Lower value"=21, "Upper value"=150}, "Blue or Luma or Val or Inten Range"={"Lower value"=147, "Upper value"=225}}, {"Red or Hue Range"={"Lower value"=0, "Upper value"=255}, "Green or Sat Range"={"Lower value"=55, "Upper value"=207}, "Blue or Luma or Val or Inten Range"={"Lower value"=163, "Upper value"=239}}, {"Red or Hue Range"={"Lower value"=0, "Upper value"=255}, "Green or Sat Range"={"Lower value"=50, "Upper value"=203}, "Blue or Luma or Val or Inten Range"={"Lower value"=159, "Upper value"=238}}, {"Red or Hue Range"={"Lower value"=0, "Upper value"=255}, "Green or Sat Range"={"Lower value"=47, "Upper value"=207}, "Blue or Luma or Val or Inten Range"={"Lower value"=162, "Upper value"=240}}, {"Red or Hue Range"={"Lower value"=0, "Upper value"=255}, "Green or Sat Range"={"Lower value"=53, "Upper value"=205}, "Blue or Luma or Val or Inten Range"={"Lower value"=160, "Upper value"=239}}, {"Red or Hue Range"={"Lower value"=0, "Upper value"=255}, "Green or Sat Range"={"Lower value"=47, "Upper value"=212}, "Blue or Luma or Val or Inten Range"={"Lower value"=160, "Upper value"=242}}, {"Red or Hue Range"={"Lower value"=0, "Upper value"=255}, "Green or Sat Range"={"Lower value"=47, "Upper value"=202}, "Blue or Luma or Val or Inten Range"={"Lower value"=160, "Upper value"=238}}, {"Red or Hue Range"={"Lower value"=0, "Upper value"=255}, "Green or Sat Range"={"Lower value"=47, "Upper value"=207}, "Blue or Luma or Val or Inten Range"={"Lower value"=161, "Upper value"=239}}, {"Red or Hue Range"={"Lower value"=0, "Upper value"=255}, "Green or Sat Range"={"Lower value"=52, "Upper value"=224}, "Blue or Luma or Val or Inten Range"={"Lower value"=163, "Upper value"=246}}, {"Red or Hue Range"={"Lower value"=0, "Upper value"=255}, "Green or Sat Range"={"Lower value"=48, "Upper value"=224}, "Blue or Luma or Val or Inten Range"={"Lower value"=156, "Upper value"=246}}, {"Red or Hue Range"={"Lower value"=0, "Upper value"=255}, "Green or Sat Range"={"Lower value"=54, "Upper value"=207}, "Blue or Luma or Val or Inten Range"={"Lower value"=163, "Upper value"=240}}, {"Red or Hue Range"={"Lower value"=0, "Upper value"=255}, "Green or Sat Range"={"Lower value"=57, "Upper value"=212}, "Blue or Luma or Val or Inten Range"={"Lower value"=162, "Upper value"=241}}, {"Red or Hue Range"={"Lower value"=0, "Upper value"=255}, "Green or Sat Range"={"Lower value"=50, "Upper value"=225}, "Blue or Luma or Val or Inten Range"={"Lower value"=164, "Upper value"=246}}, {"Red or Hue Range"={"Lower value"=0, "Upper value"=255}, "Green or Sat Range"={"Lower value"=48, "Upper value"=208}, "Blue or Luma or Val or Inten Range"={"Lower value"=157, "Upper value"=240}}, {"Red or Hue Range"={"Lower value"=0, "Upper value"=255}, "Green or Sat Range"={"Lower value"=48, "Upper value"=199}, "Blue or Luma or Val or Inten Range"={"Lower value"=165, "Upper value"=236}}, {"Red or Hue Range"={"Lower value"=0, "Upper value"=255}, "Green or Sat Range"={"Lower value"=53, "Upper value"=207}, "Blue or Luma or Val or Inten Range"={"Lower value"=161, "Upper value"=239}}, {"Red or Hue Range"={"Lower value"=0, "Upper value"=255}, "Green or Sat Range"={"Lower value"=53, "Upper value"=215}, "Blue or Luma or Val or Inten Range"={"Lower value"=155, "Upper value"=242}}, {"Red or Hue Range"={"Lower value"=0, "Upper value"=255}, "Green or Sat Range"={"Lower value"=47, "Upper value"=210}, "Blue or Luma or Val or Inten Range"={"Lower value"=164, "Upper value"=241}}, {"Red or Hue Range"={"Lower value"=0, "Upper value"=255}, "Green or Sat Range"={"Lower value"=0, "Upper value"=255}, "Blue or Luma or Val or Inten Range"={"Lower value"=60, "Upper value"=255}}, {"Red or Hue Range"={"Lower value"=0, "Upper value"=255}, "Green or Sat Range"={"Lower value"=0, "Upper value"=255}, "Blue or Luma or Val or Inten Range"={"Lower value"=60, "Upper value"=255}}, {"Red or Hue Range"={"Lower value"=0, "Upper value"=255}, "Green or Sat Range"={"Lower value"=0, "Upper value"=255}, "Blue or Luma or Val or Inten Range"={"Lower value"=61, "Upper value"=255}}, {"Red or Hue Range"={"Lower value"=0, "Upper value"=255}, "Green or Sat Range"={"Lower value"=0, "Upper value"=255}, "Blue or Luma or Val or Inten Range"={"Lower value"=60, "Upper value"=255}}, {"Red or Hue Range"={"Lower value"=0, "Upper value"=255}, "Green or Sat Range"={"Lower value"=0, "Upper value"=255}, "Blue or Luma or Val or Inten Range"={"Lower value"=110, "Upper value"=255}}, {"Red or Hue Range"={"Lower value"=0, "Upper value"=255}, "Green or Sat Range"={"Lower value"=0, "Upper value"=255}, "Blue or Luma or Val or Inten Range"={"Lower value"=108, "Upper value"=255}}, {"Red or Hue Range"={"Lower value"=0, "Upper value"=255}, "Green or Sat Range"={"Lower value"=0, "Upper value"=255}, "Blue or Luma or Val or Inten Range"={"Lower value"=108, "Upper value"=255}}, {"Red or Hue Range"={"Lower value"=0, "Upper value"=255}, "Green or Sat Range"={"Lower value"=0, "Upper value"=255}, "Blue or Luma or Val or Inten Range"={"Lower value"=106, "Upper value"=255}}, {"Red or Hue Range"={"Lower value"=0, "Upper value"=255}, "Green or Sat Range"={"Lower value"=0, "Upper value"=255}, "Blue or Luma or Val or Inten Range"={"Lower value"=108, "Upper value"=255}}, {"Red or Hue Range"={"Lower value"=0, "Upper value"=255}, "Green or Sat Range"={"Lower value"=0, "Upper value"=255}, "Blue or Luma or Val or Inten Range"={"Lower value"=107, "Upper value"=255}}, {"Red or Hue Range"={"Lower value"=0, "Upper value"=255}, "Green or Sat Range"={"Lower value"=0, "Upper value"=255}, "Blue or Luma or Val or Inten Range"={"Lower value"=106, "Upper value"=255}}, {"Red or Hue Range"={"Lower value"=0, "Upper value"=255}, "Green or Sat Range"={"Lower value"=0, "Upper value"=255}, "Blue or Luma or Val or Inten Range"={"Lower value"=109, "Upper value"=255}}, {"Red or Hue Range"={"Lower value"=0, "Upper value"=255}, "Green or Sat Range"={"Lower value"=0, "Upper value"=255}, "Blue or Luma or Val or Inten Range"={"Lower value"=109, "Upper value"=255}}, {"Red or Hue Range"={"Lower value"=0, "Upper value"=255}, "Green or Sat Range"={"Lower value"=0, "Upper value"=255}, "Blue or Luma or Val or Inten Range"={"Lower value"=109, "Upper value"=255}}, {"Red or Hue Range"={"Lower value"=0, "Upper value"=255}, "Green or Sat Range"={"Lower value"=0, "Upper value"=255}, "Blue or Luma or Val or Inten Range"={"Lower value"=109, "Upper value"=255}}, {"Red or Hue Range"={"Lower value"=0, "Upper value"=255}, "Green or Sat Range"={"Lower value"=0, "Upper value"=255}, "Blue or Luma or Val or Inten Range"={"Lower value"=106, "Upper value"=255}}, {"Red or Hue Range"={"Lower value"=0, "Upper value"=255}, "Green or Sat Range"={"Lower value"=0, "Upper value"=255}, "Blue or Luma or Val or Inten Range"={"Lower value"=108, "Upper value"=255}}, {"Red or Hue Range"={"Lower value"=0, "Upper value"=255}, "Green or Sat Range"={"Lower value"=0, "Upper value"=255}, "Blue or Luma or Val or Inten Range"={"Lower value"=110, "Upper value"=255}}, {"Red or Hue Range"={"Lower value"=0, "Upper value"=255}, "Green or Sat Range"={"Lower value"=238, "Upper value"=255}, "Blue or Luma or Val or Inten Range"={"Lower value"=249, "Upper value"=255}}, {"Red or Hue Range"={"Lower value"=0, "Upper value"=255}, "Green or Sat Range"={"Lower value"=244, "Upper value"=255}, "Blue or Luma or Val or Inten Range"={"Lower value"=251, "Upper value"=255}}, {"Red or Hue Range"={"Lower value"=0, "Upper value"=255}, "Green or Sat Range"={"Lower value"=226, "Upper value"=255}, "Blue or Luma or Val or Inten Range"={"Lower value"=245, "Upper value"=255}}, {"Red or Hue Range"={"Lower value"=0, "Upper value"=255}, "Green or Sat Range"={"Lower value"=240, "Upper value"=255}, "Blue or Luma or Val or Inten Range"={"Lower value"=250, "Upper value"=255}}, {"Red or Hue Range"={"Lower value"=0, "Upper value"=255}, "Green or Sat Range"={"Lower value"=234, "Upper value"=255}, "Blue or Luma or Val or Inten Range"={"Lower value"=248, "Upper value"=255}}, {"Red or Hue Range"={"Lower value"=0, "Upper value"=255}, "Green or Sat Range"={"Lower value"=229, "Upper value"=255}, "Blue or Luma or Val or Inten Range"={"Lower value"=246, "Upper value"=255}}, {"Red or Hue Range"={"Lower value"=0, "Upper value"=255}, "Green or Sat Range"={"Lower value"=228, "Upper value"=255}, "Blue or Luma or Val or Inten Range"={"Lower value"=246, "Upper value"=255}}, {"Red or Hue Range"={"Lower value"=0, "Upper value"=255}, "Green or Sat Range"={"Lower value"=233, "Upper value"=255}, "Blue or Luma or Val or Inten Range"={"Lower value"=246, "Upper value"=255}}, {"Red or Hue Range"={"Lower value"=0, "Upper value"=255}, "Green or Sat Range"={"Lower value"=233, "Upper value"=255}, "Blue or Luma or Val or Inten Range"={"Lower value"=247, "Upper value"=255}}, {"Red or Hue Range"={"Lower value"=0, "Upper value"=255}, "Green or Sat Range"={"Lower value"=240, "Upper value"=255}, "Blue or Luma or Val or Inten Range"={"Lower value"=249, "Upper value"=255}}, {"Red or Hue Range"={"Lower value"=0, "Upper value"=255}, "Green or Sat Range"={"Lower value"=233, "Upper value"=255}, "Blue or Luma or Val or Inten Range"={"Lower value"=247, "Upper value"=255}}, {"Red or Hue Range"={"Lower value"=0, "Upper value"=255}, "Green or Sat Range"={"Lower value"=230, "Upper value"=255}, "Blue or Luma or Val or Inten Range"={"Lower value"=245, "Upper value"=255}}, {"Red or Hue Range"={"Lower value"=0, "Upper value"=255}, "Green or Sat Range"={"Lower value"=225, "Upper value"=255}, "Blue or Luma or Val or Inten Range"={"Lower value"=243, "Upper value"=255}}, {"Red or Hue Range"={"Lower value"=0, "Upper value"=255}, "Green or Sat Range"={"Lower value"=233, "Upper value"=255}, "Blue or Luma or Val or Inten Range"={"Lower value"=247, "Upper value"=255}}, {"Red or Hue Range"={"Lower value"=0, "Upper value"=255}, "Green or Sat Range"={"Lower value"=231, "Upper value"=255}, "Blue or Luma or Val or Inten Range"={"Lower value"=247, "Upper value"=255}}, {"Red or Hue Range"={"Lower value"=0, "Upper value"=255}, "Green or Sat Range"={"Lower value"=225, "Upper value"=255}, "Blue or Luma or Val or Inten Range"={"Lower value"=243, "Upper value"=255}}, {"Red or Hue Range"={"Lower value"=0, "Upper value"=255}, "Green or Sat Range"={"Lower value"=227, "Upper value"=255}, "Blue or Luma or Val or Inten Range"={"Lower value"=244, "Upper value"=255}}, {"Red or Hue Range"={"Lower value"=0, "Upper value"=255}, "Green or Sat Range"={"Lower value"=225, "Upper value"=255}, "Blue or Luma or Val or Inten Range"={"Lower value"=244, "Upper value"=255}}, {"Red or Hue Range"={"Lower value"=0, "Upper value"=255}, "Green or Sat Range"={"Lower value"=222, "Upper value"=255}, "Blue or Luma or Val or Inten Range"={"Lower value"=244, "Upper value"=255}}, {"Red or Hue Range"={"Lower value"=0, "Upper value"=255}, "Green or Sat Range"={"Lower value"=235, "Upper value"=255}, "Blue or Luma or Val or Inten Range"={"Lower value"=247, "Upper value"=255}}, {"Red or Hue Range"={"Lower value"=0, "Upper value"=255}, "Green or Sat Range"={"Lower value"=223, "Upper value"=255}, "Blue or Luma or Val or Inten Range"={"Lower value"=243, "Upper value"=255}}, {"Red or Hue Range"={"Lower value"=0, "Upper value"=255}, "Green or Sat Range"={"Lower value"=212, "Upper value"=255}, "Blue or Luma or Val or Inten Range"={"Lower value"=237, "Upper value"=255}}, {"Red or Hue Range"={"Lower value"=0, "Upper value"=255}, "Green or Sat Range"={"Lower value"=205, "Upper value"=255}, "Blue or Luma or Val or Inten Range"={"Lower value"=234, "Upper value"=255}}, {"Red or Hue Range"={"Lower value"=0, "Upper value"=255}, "Green or Sat Range"={"Lower value"=211, "Upper value"=255}, "Blue or Luma or Val or Inten Range"={"Lower value"=235, "Upper value"=255}}, {"Red or Hue Range"={"Lower value"=0, "Upper value"=255}, "Green or Sat Range"={"Lower value"=211, "Upper value"=255}, "Blue or Luma or Val or Inten Range"={"Lower value"=236, "Upper value"=255}}, {"Red or Hue Range"={"Lower value"=0, "Upper value"=255}, "Green or Sat Range"={"Lower value"=212, "Upper value"=255}, "Blue or Luma or Val or Inten Range"={"Lower value"=237, "Upper value"=255}}, {"Red or Hue Range"={"Lower value"=0, "Upper value"=255}, "Green or Sat Range"={"Lower value"=206, "Upper value"=255}, "Blue or Luma or Val or Inten Range"={"Lower value"=234, "Upper value"=255}}, {"Red or Hue Range"={"Lower value"=0, "Upper value"=255}, "Green or Sat Range"={"Lower value"=217, "Upper value"=255}, "Blue or Luma or Val or Inten Range"={"Lower value"=239, "Upper value"=255}}, {"Red or Hue Range"={"Lower value"=0, "Upper value"=255}, "Green or Sat Range"={"Lower value"=206, "Upper value"=255}, "Blue or Luma or Val or Inten Range"={"Lower value"=234, "Upper value"=255}}, {"Red or Hue Range"={"Lower value"=0, "Upper value"=255}, "Green or Sat Range"={"Lower value"=212, "Upper value"=255}, "Blue or Luma or Val or Inten Range"={"Lower value"=237, "Upper value"=255}}, {"Red or Hue Range"={"Lower value"=0, "Upper value"=255}, "Green or Sat Range"={"Lower value"=214, "Upper value"=255}, "Blue or Luma or Val or Inten Range"={"Lower value"=238, "Upper value"=255}}, {"Red or Hue Range"={"Lower value"=0, "Upper value"=255}, "Green or Sat Range"={"Lower value"=210, "Upper value"=255}, "Blue or Luma or Val or Inten Range"={"Lower value"=236, "Upper value"=255}}, {"Red or Hue Range"={"Lower value"=0, "Upper value"=255}, "Green or Sat Range"={"Lower value"=212, "Upper value"=255}, "Blue or Luma or Val or Inten Range"={"Lower value"=237, "Upper value"=255}}, {"Red or Hue Range"={"Lower value"=0, "Upper value"=255}, "Green or Sat Range"={"Lower value"=212, "Upper value"=255}, "Blue or Luma or Val or Inten Range"={"Lower value"=237, "Upper value"=255}}, {"Red or Hue Range"={"Lower value"=0, "Upper value"=255}, "Green or Sat Range"={"Lower value"=203, "Upper value"=255}, "Blue or Luma or Val or Inten Range"={"Lower value"=233, "Upper value"=255}}, {"Red or Hue Range"={"Lower value"=0, "Upper value"=255}, "Green or Sat Range"={"Lower value"=207, "Upper value"=255}, "Blue or Luma or Val or Inten Range"={"Lower value"=228, "Upper value"=255}}, {"Red or Hue Range"={"Lower value"=0, "Upper value"=255}, "Green or Sat Range"={"Lower value"=216, "Upper value"=255}, "Blue or Luma or Val or Inten Range"={"Lower value"=239, "Upper value"=255}}, {"Red or Hue Range"={"Lower value"=0, "Upper value"=255}, "Green or Sat Range"={"Lower value"=214, "Upper value"=255}, "Blue or Luma or Val or Inten Range"={"Lower value"=238, "Upper value"=255}}, {"Red or Hue Range"={"Lower value"=0, "Upper value"=255}, "Green or Sat Range"={"Lower value"=206, "Upper value"=255}, "Blue or Luma or Val or Inten Range"={"Lower value"=234, "Upper value"=255}}, {"Red or Hue Range"={"Lower value"=0, "Upper value"=255}, "Green or Sat Range"={"Lower value"=211, "Upper value"=255}, "Blue or Luma or Val or Inten Range"={"Lower value"=237, "Upper value"=255}}, {"Red or Hue Range"={"Lower value"=0, "Upper value"=255}, "Green or Sat Range"={"Lower value"=207, "Upper value"=255}, "Blue or Luma or Val or Inten Range"={"Lower value"=231, "Upper value"=255}}, {"Red or Hue Range"={"Lower value"=0, "Upper value"=255}, "Green or Sat Range"={"Lower value"=212, "Upper value"=255}, "Blue or Luma or Val or Inten Range"={"Lower value"=237, "Upper value"=255}}, {"Red or Hue Range"={"Lower value"=0, "Upper value"=255}, "Green or Sat Range"={"Lower value"=210, "Upper value"=255}, "Blue or Luma or Val or Inten Range"={"Lower value"=236, "Upper value"=255}}, {"Red or Hue Range"={"Lower value"=0, "Upper value"=255}, "Green or Sat Range"={"Lower value"=214, "Upper value"=255}, "Blue or Luma or Val or Inten Range"={"Lower value"=238, "Upper value"=255}}, {"Red or Hue Range"={"Lower value"=0, "Upper value"=255}, "Green or Sat Range"={"Lower value"=212, "Upper value"=255}, "Blue or Luma or Val or Inten Range"={"Lower value"=236, "Upper value"=255}}, {"Red or Hue Range"={"Lower value"=0, "Upper value"=255}, "Green or Sat Range"={"Lower value"=205, "Upper value"=255}, "Blue or Luma or Val or Inten Range"={"Lower value"=234, "Upper value"=255}}, {"Red or Hue Range"={"Lower value"=0, "Upper value"=255}, "Green or Sat Range"={"Lower value"=53, "Upper value"=255}, "Blue or Luma or Val or Inten Range"={"Lower value"=163, "Upper value"=255}}, {"Red or Hue Range"={"Lower value"=0, "Upper value"=255}, "Green or Sat Range"={"Lower value"=47, "Upper value"=255}, "Blue or Luma or Val or Inten Range"={"Lower value"=163, "Upper value"=255}}, {"Red or Hue Range"={"Lower value"=0, "Upper value"=255}, "Green or Sat Range"={"Lower value"=57, "Upper value"=255}, "Blue or Luma or Val or Inten Range"={"Lower value"=163, "Upper value"=255}}, {"Red or Hue Range"={"Lower value"=0, "Upper value"=255}, "Green or Sat Range"={"Lower value"=51, "Upper value"=255}, "Blue or Luma or Val or Inten Range"={"Lower value"=166, "Upper value"=255}}, {"Red or Hue Range"={"Lower value"=0, "Upper value"=255}, "Green or Sat Range"={"Lower value"=54, "Upper value"=255}, "Blue or Luma or Val or Inten Range"={"Lower value"=167, "Upper value"=255}}, {"Red or Hue Range"={"Lower value"=0, "Upper value"=255}, "Green or Sat Range"={"Lower value"=59, "Upper value"=255}, "Blue or Luma or Val or Inten Range"={"Lower value"=166, "Upper value"=255}}, {"Red or Hue Range"={"Lower value"=0, "Upper value"=255}, "Green or Sat Range"={"Lower value"=49, "Upper value"=255}, "Blue or Luma or Val or Inten Range"={"Lower value"=162, "Upper value"=255}}, {"Red or Hue Range"={"Lower value"=0, "Upper value"=255}, "Green or Sat Range"={"Lower value"=53, "Upper value"=255}, "Blue or Luma or Val or Inten Range"={"Lower value"=166, "Upper value"=255}}, {"Red or Hue Range"={"Lower value"=0, "Upper value"=255}, "Green or Sat Range"={"Lower value"=57, "Upper value"=255}, "Blue or Luma or Val or Inten Range"={"Lower value"=167, "Upper value"=255}}, {"Red or Hue Range"={"Lower value"=0, "Upper value"=255}, "Green or Sat Range"={"Lower value"=54, "Upper value"=255}, "Blue or Luma or Val or Inten Range"={"Lower value"=164, "Upper value"=255}}, {"Red or Hue Range"={"Lower value"=0, "Upper value"=255}, "Green or Sat Range"={"Lower value"=56, "Upper value"=255}, "Blue or Luma or Val or Inten Range"={"Lower value"=168, "Upper value"=255}}, {"Red or Hue Range"={"Lower value"=0, "Upper value"=255}, "Green or Sat Range"={"Lower value"=52, "Upper value"=255}, "Blue or Luma or Val or Inten Range"={"Lower value"=167, "Upper value"=255}}, {"Red or Hue Range"={"Lower value"=0, "Upper value"=255}, "Green or Sat Range"={"Lower value"=52, "Upper value"=255}, "Blue or Luma or Val or Inten Range"={"Lower value"=166, "Upper value"=255}}, {"Red or Hue Range"={"Lower value"=0, "Upper value"=255}, "Green or Sat Range"={"Lower value"=55, "Upper value"=255}, "Blue or Luma or Val or Inten Range"={"Lower value"=164, "Upper value"=255}}, {"Red or Hue Range"={"Lower value"=0, "Upper value"=255}, "Green or Sat Range"={"Lower value"=53, "Upper value"=255}, "Blue or Luma or Val or Inten Range"={"Lower value"=165, "Upper value"=255}}, {"Red or Hue Range"={"Lower value"=0, "Upper value"=255}, "Green or Sat Range"={"Lower value"=46, "Upper value"=255}, "Blue or Luma or Val or Inten Range"={"Lower value"=163, "Upper value"=255}}, {"Red or Hue Range"={"Lower value"=0, "Upper value"=255}, "Green or Sat Range"={"Lower value"=56, "Upper value"=255}, "Blue or Luma or Val or Inten Range"={"Lower value"=167, "Upper value"=255}}, {"Red or Hue Range"={"Lower value"=0, "Upper value"=255}, "Green or Sat Range"={"Lower value"=56, "Upper value"=255}, "Blue or Luma or Val or Inten Range"={"Lower value"=166, "Upper value"=255}}, {"Red or Hue Range"={"Lower value"=0, "Upper value"=255}, "Green or Sat Range"={"Lower value"=48, "Upper value"=255}, "Blue or Luma or Val or Inten Range"={"Lower value"=164, "Upper value"=255}}, {"Red or Hue Range"={"Lower value"=0, "Upper value"=255}, "Green or Sat Range"={"Lower value"=45, "Upper value"=255}, "Blue or Luma or Val or Inten Range"={"Lower value"=161, "Upper value"=255}}, {"Red or Hue Range"={"Lower value"=0, "Upper value"=255}, "Green or Sat Range"={"Lower value"=60, "Upper value"=255}, "Blue or Luma or Val or Inten Range"={"Lower value"=169, "Upper value"=255}}, {"Red or Hue Range"={"Lower value"=0, "Upper value"=255}, "Green or Sat Range"={"Lower value"=55, "Upper value"=255}, "Blue or Luma or Val or Inten Range"={"Lower value"=165, "Upper value"=255}}, {"Red or Hue Range"={"Lower value"=0, "Upper value"=255}, "Green or Sat Range"={"Lower value"=50, "Upper value"=255}, "Blue or Luma or Val or Inten Range"={"Lower value"=164, "Upper value"=255}}, {"Red or Hue Range"={"Lower value"=0, "Upper value"=255}, "Green or Sat Range"={"Lower value"=51, "Upper value"=255}, "Blue or Luma or Val or Inten Range"={"Lower value"=164, "Upper value"=255}}, {"Red or Hue Range"={"Lower value"=0, "Upper value"=255}, "Green or Sat Range"={"Lower value"=59, "Upper value"=255}, "Blue or Luma or Val or Inten Range"={"Lower value"=167, "Upper value"=255}}, {"Red or Hue Range"={"Lower value"=0, "Upper value"=255}, "Green or Sat Range"={"Lower value"=49, "Upper value"=255}, "Blue or Luma or Val or Inten Range"={"Lower value"=163, "Upper value"=255}}, {"Red or Hue Range"={"Lower value"=0, "Upper value"=255}, "Green or Sat Range"={"Lower value"=51, "Upper value"=255}, "Blue or Luma or Val or Inten Range"={"Lower value"=165, "Upper value"=255}}, {"Red or Hue Range"={"Lower value"=0, "Upper value"=255}, "Green or Sat Range"={"Lower value"=52, "Upper value"=255}, "Blue or Luma or Val or Inten Range"={"Lower value"=164, "Upper value"=255}}, {"Red or Hue Range"={"Lower value"=0, "Upper value"=255}, "Green or Sat Range"={"Lower value"=52, "Upper value"=255}, "Blue or Luma or Val or Inten Range"={"Lower value"=167, "Upper value"=255}}, {"Red or Hue Range"={"Lower value"=0, "Upper value"=255}, "Green or Sat Range"={"Lower value"=54, "Upper value"=255}, "Blue or Luma or Val or Inten Range"={"Lower value"=167, "Upper value"=255}}, {"Red or Hue Range"={"Lower value"=0, "Upper value"=255}, "Green or Sat Range"={"Lower value"=47, "Upper value"=255}, "Blue or Luma or Val or Inten Range"={"Lower value"=164, "Upper value"=255}}, {"Red or Hue Range"={"Lower value"=0, "Upper value"=255}, "Green or Sat Range"={"Lower value"=53, "Upper value"=255}, "Blue or Luma or Val or Inten Range"={"Lower value"=167, "Upper value"=255}}, {"Red or Hue Range"={"Lower value"=0, "Upper value"=255}, "Green or Sat Range"={"Lower value"=51, "Upper value"=255}, "Blue or Luma or Val or Inten Range"={"Lower value"=167, "Upper value"=255}}, {"Red or Hue Range"={"Lower value"=0, "Upper value"=255}, "Green or Sat Range"={"Lower value"=49, "Upper value"=255}, "Blue or Luma or Val or Inten Range"={"Lower value"=163, "Upper value"=255}}, {"Red or Hue Range"={"Lower value"=0, "Upper value"=255}, "Green or Sat Range"={"Lower value"=50, "Upper value"=255}, "Blue or Luma or Val or Inten Range"={"Lower value"=168, "Upper value"=255}}, {"Red or Hue Range"={"Lower value"=0, "Upper value"=255}, "Green or Sat Range"={"Lower value"=54, "Upper value"=255}, "Blue or Luma or Val or Inten Range"={"Lower value"=166, "Upper value"=255}}, {"Red or Hue Range"={"Lower value"=0, "Upper value"=255}, "Green or Sat Range"={"Lower value"=53, "Upper value"=255}, "Blue or Luma or Val or Inten Range"={"Lower value"=168, "Upper value"=255}}, {"Red or Hue Range"={"Lower value"=0, "Upper value"=255}, "Green or Sat Range"={"Lower value"=47, "Upper value"=255}, "Blue or Luma or Val or Inten Range"={"Lower value"=163, "Upper value"=255}}, {"Red or Hue Range"={"Lower value"=0, "Upper value"=255}, "Green or Sat Range"={"Lower value"=52, "Upper value"=255}, "Blue or Luma or Val or Inten Range"={"Lower value"=166, "Upper value"=255}}, {"Red or Hue Range"={"Lower value"=0, "Upper value"=255}, "Green or Sat Range"={"Lower value"=53, "Upper value"=255}, "Blue or Luma or Val or Inten Range"={"Lower value"=169, "Upper value"=255}}, {"Red or Hue Range"={"Lower value"=0, "Upper value"=255}, "Green or Sat Range"={"Lower value"=50, "Upper value"=255}, "Blue or Luma or Val or Inten Range"={"Lower value"=164, "Upper value"=255}}, {"Red or Hue Range"={"Lower value"=0, "Upper value"=255}, "Green or Sat Range"={"Lower value"=48, "Upper value"=255}, "Blue or Luma or Val or Inten Range"={"Lower value"=165, "Upper value"=255}}]
  out "color element":T10
  out "Particle":T11(plugin-control)
  out "Particle 2":T11(plugin-control)
  out "Particle 3":T11(plugin-control)
  in  "Color Sampling":bool
  in  "Color Index":i32
  out "Color":T11(plugin-control)
  in  "Mode":enum16{"Camera Off", "Camera On", "Scan QR"}(ring)
  in  "stop":bool
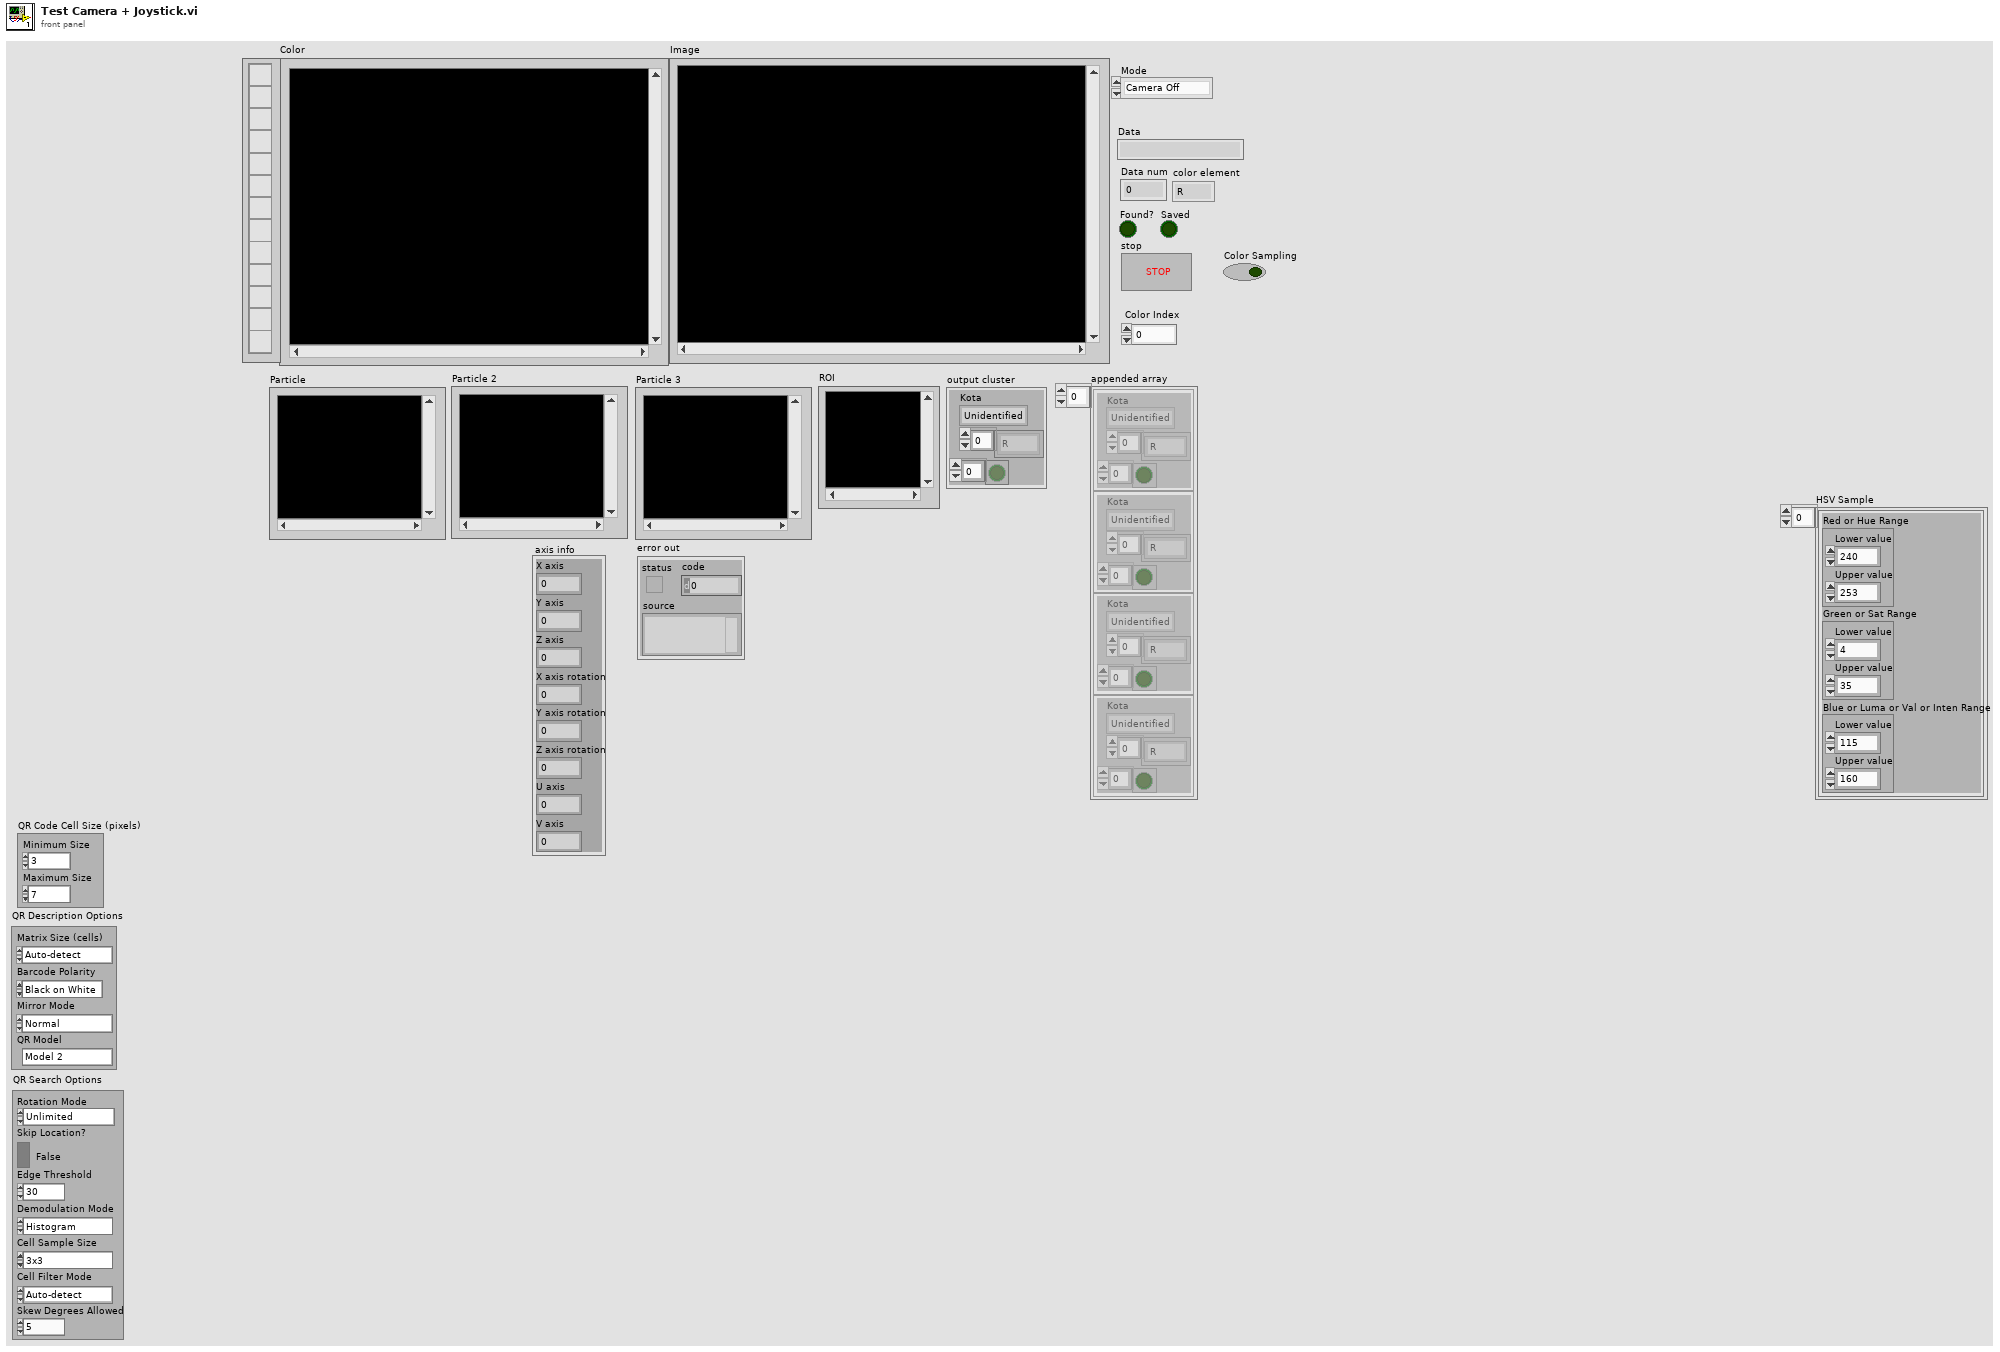
[diagram p1: front panel]
types:
  T1 = cluster{"X axis":i32, "Y axis":i32, "Z axis":i32, "X axis rotation":i32, "Y axis rotation":i32, "Z axis rotation":i32, "U axis":i32, "V axis":i32}
  T2 = typedef "QR Code Description Options.ctl" = cluster{"Matrix Size (cells)":i32, "Barcode Polarity":T3, "Mirror Mode":i32, "QR Model":T4}
  T3 = typedef "Data Matrix Polarity.ctl" = i32
  T4 = typedef "QR Code Model Type.ctl" = i32
  T5 = typedef "QR Code Search Options.ctl" = cluster{"Rotation Mode":enum32{"Unlimited", "0 Degrees", "90 Degrees", "180 Degrees", "270 Degrees"}, "Skip Location?":bool, "Edge Threshold":u32, "Demodulation Mode":T6, "Cell Sample Size":T7, "Cell Filter Mode":T8, "Skew Degrees Allowed":u32}
  T6 = typedef "Demodulation Mode.ctl" = i32
  T7 = typedef "Cell Sample Size.ctl" = i32
  T8 = typedef "Cell Filter Mode.ctl" = i32
  T9 = typedef "Kota.ctl" = enum16{"Unidentified", "1", "2", "3", "4"}
  T10 = typedef "Barang.ctl" = enum16{"R", "G", "B", "Y", "K"}
  T11 = typedef "IMAQ Image.ctl" = refnum<image>
  T12 = cluster{"Red or Hue Range":cluster{"Lower value":i32, "Upper value":i32}, "Green or Sat Range":cluster{"Lower value":i32, "Upper value":i32}, "Blue or Luma or Val or Inten Range":cluster{"Lower value":i32, "Upper value":i32}}[]
  T13 = typedef "IMAQdx.ctl" = refnum<k21>
  T14 = cluster{"Global Rectangle":i32[], "Contours":cluster{"Contour Type":u32, "ROI Type":u32, "Points":i32[]}[]}
  T15 = cluster{"Red or Hue Range":cluster{"Lower value":i32, "Upper value":i32}, "Green or Sat Range":cluster{"Lower value":i32, "Upper value":i32}, "Blue or Luma or Val or Inten Range":cluster{"Lower value":i32, "Upper value":i32}}
  T16 = cluster{"Area":dbl, "Number of Holes":dbl, "Bounding Rect":cluster{"Left":dbl, "Top":dbl, "Right":dbl, "Bottom":dbl}, "Center of Mass":cluster{"X":dbl, "Y":dbl}, "Orientation":dbl, "Dimensions":cluster{"Width":dbl, "Height":dbl}}[]
  T17 = cluster{"Area":dbl, "Number of Holes":dbl, "Bounding Rect":cluster{"Left":dbl, "Top":dbl, "Right":dbl, "Bottom":dbl}, "Center of Mass":cluster{"X":dbl, "Y":dbl}, "Orientation":dbl, "Dimensions":cluster{"Width":dbl, "Height":dbl}}
  T18 = cluster{"histogram":u32[], "Minimal Value":sgl, "Maximal Value":sgl, "Starting Value":sgl, "Interval Width":sgl, "Mean Value":sgl, "Standard  Variation":sgl, "Area (pixels)":i32}
  T19 = cluster{cluster{i32, i32}, cluster{i32, i32}, cluster{i32, i32}}
  T20 = typedef "QR Code Report.ctl" = cluster{"Found?":bool, "Data":string, "Bounding Box":cluster{"x":sgl, "y":sgl}[], "Errors Corrected":u32, "Dimensions (Rows/Cols)":u32, "Version":u32, "QR Model":T4, "Stream Mode":T21, "Barcode Polarity":T3, "Mirrored?":bool, "Append Stream Position":u32, "Size of Append Stream":u32, "First EAN-128 ID":i32, "First Alternate Language ID":i32, "Append Stream ID":u32, "Minimum Edge Strength":u32, "Demodulation Mode":T6, "Cell Sample Size":T7, "Cell Filter Mode":T8}
  T21 = typedef "QR Code Stream Mode Type.ctl" = i32
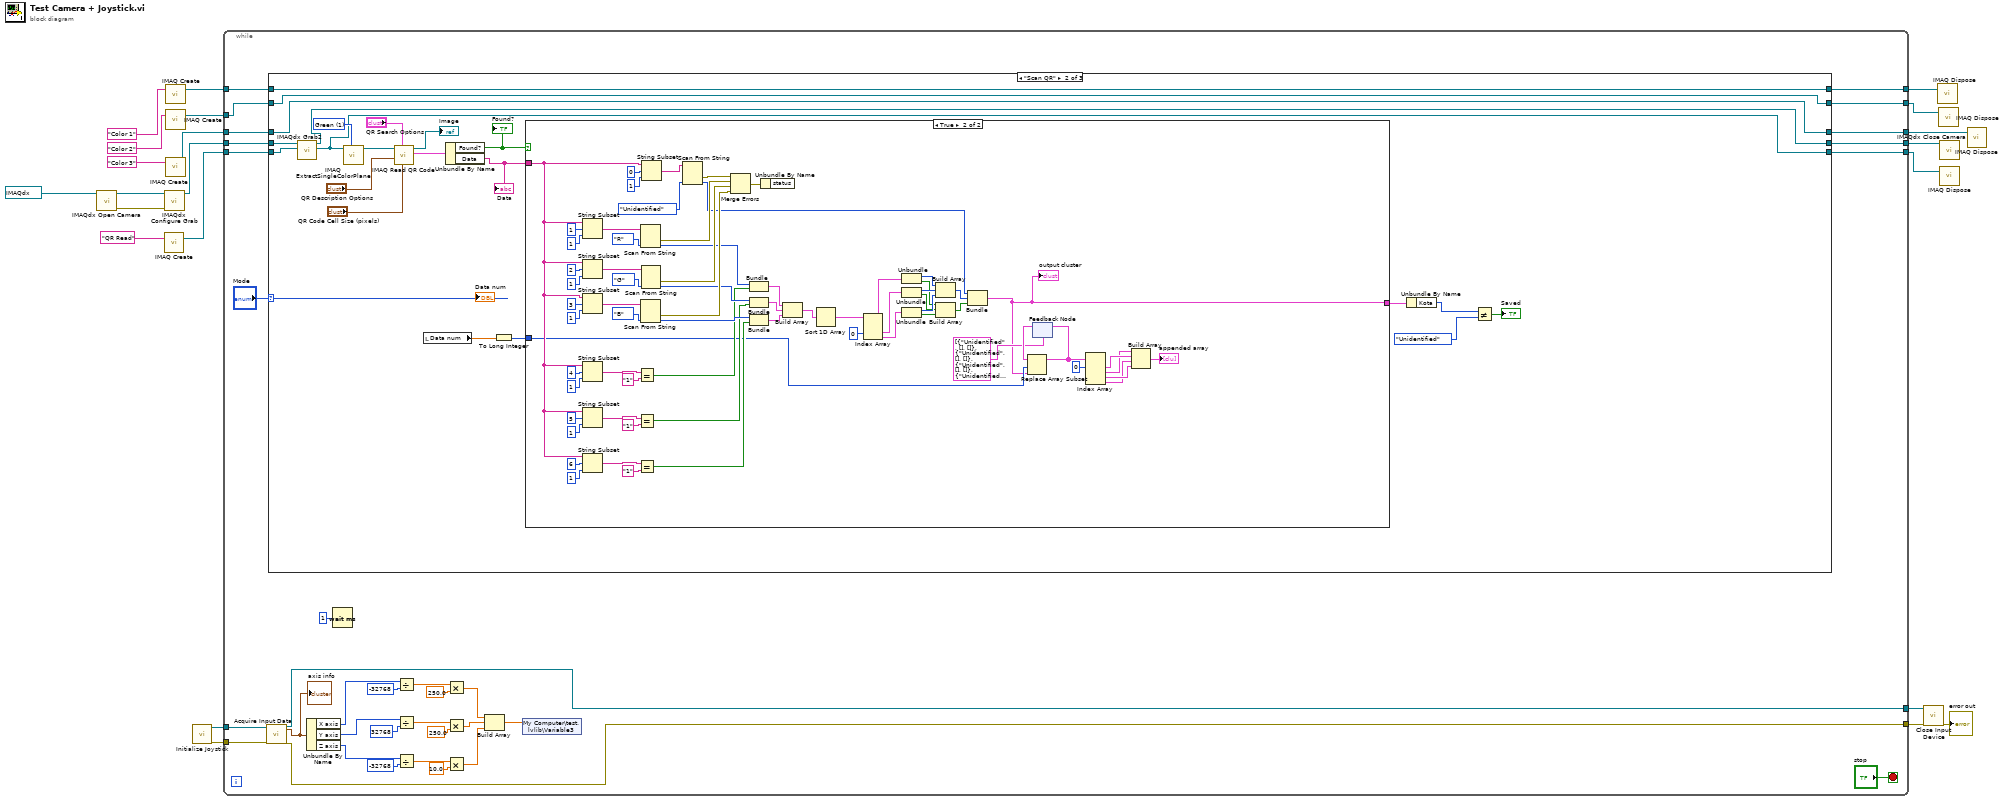
[diagram p0: block diagram]
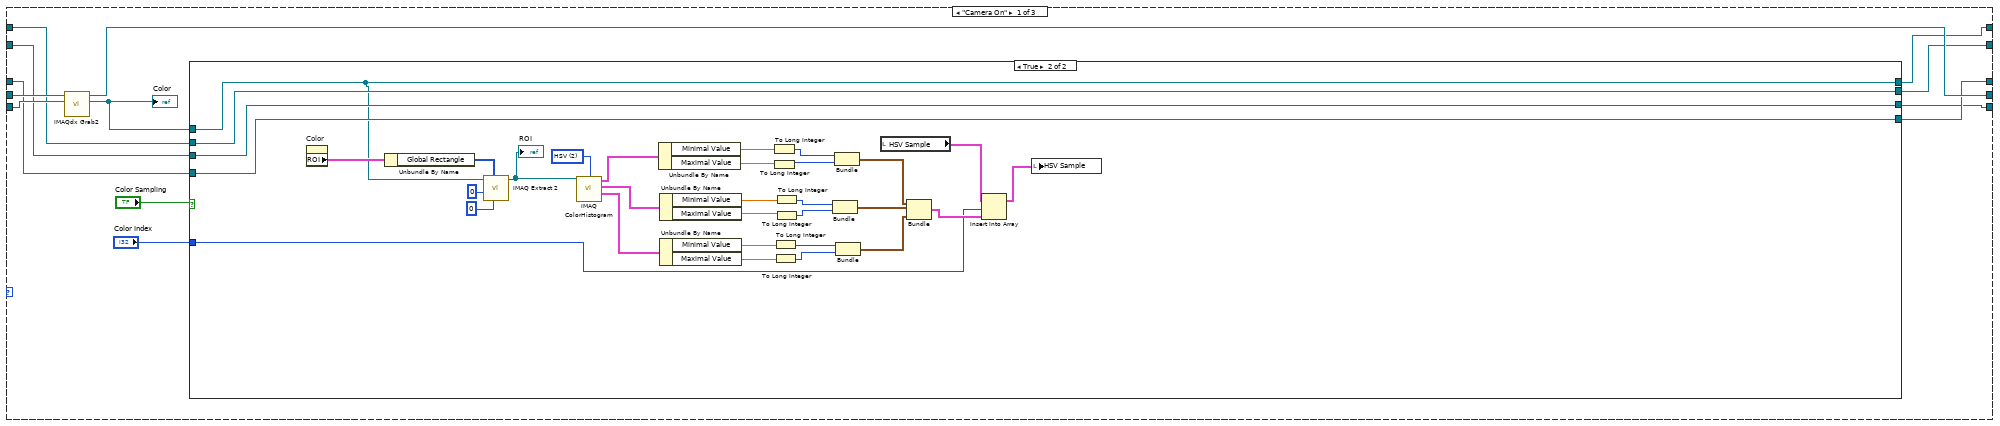
[diagram p2: hidden frame]
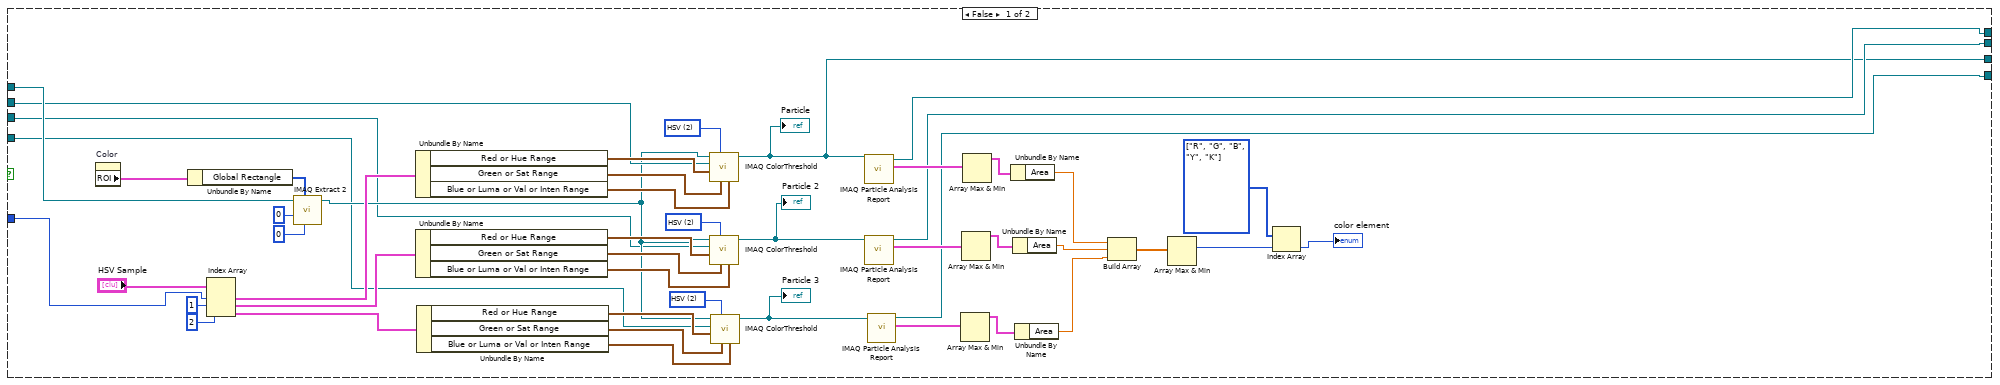
[diagram p3: hidden frame]
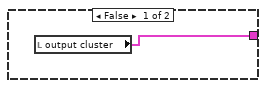
[diagram p4: hidden frame]
diagram:
  n1 = call <vilib>:"IMAQdx Open Camera.vi"("Session In"=T13 "cam0") -> ("error out"=w22:errorcluster, "Session Out"=w21:T13)  [unwired: 9 in]
  n2 = call "IMAQ Create"("Image Name"="QR Read") -> ("New Image"=w11:T11)  [unwired: 4 in, 1 out]
  n3 = call <vilib>:"IMAQdx Configure Grab.vi"("error in"=w22, "Session In"=w21) -> ("Session Out"=w12:T13)  [unwired: 8 in, 1 out]
  n4 = call "IMAQ Create"("Image Name"="Color 1") -> ("New Image"=w15:T11)  [unwired: 4 in, 1 out]
  n5 = call "IMAQ Create"("Image Name"="Color 2") -> ("New Image"=w14:T11)  [unwired: 4 in, 1 out]
  n6 = call "IMAQ Create"("Image Name"="Color 3") -> ("New Image"=w13:T11)  [unwired: 4 in, 1 out]
  n7 = call <vilib>:"Initialize Joystick.vi"() -> ("error out"=w4:errorcluster, "device ID"=w5:refnum<k1>)  [unwired: 10 in]
  n8 = while {
    tunnel: w15 -> [w55]
    tunnel: w14 -> [w46]
    tunnel: w13 -> [w54]
    tunnel: w12 -> [w53]
    tunnel: w11 -> [w52]
    tunnel: [w51] -> w9
    tunnel: [w50] -> w8
    tunnel: [w49] -> w7
    tunnel: [w48] -> w10
    tunnel: [w47] -> w6
    tunnel: w5 -> [w44]
    tunnel: w4 -> [w43]
    tunnel: [w24] -> w3
    tunnel: [w23] -> w1
    stop <- "stop" stop-if-true
    n9 = call-poly <vilib>:"Acquire Input Data.vi"("device ID"=w44, "error in (no error)"=w43) -> ("device ID"=w24:refnum<k1>, "axis info"=w42:T1, "error out"=w23:errorcluster)  [unwired: 13 in, 2 out]
    "axis info" <- w42
    n10 = case shown="\"Scan QR\"" "Mode" {
      tunnel: w55 -> [w63 w152 w245]
      tunnel: w46 -> [w64 w151 w244]
      tunnel: w54 -> [w65 w150 w243]
      tunnel: w53 -> [w69 w169 w242]
      tunnel: w52 -> [w68 w170 w241]
      tunnel: [w58 w152 w245] -> w51
      tunnel: [w59 w151 w244] -> w50
      tunnel: [w61 w150 w243] -> w49
      tunnel: [w66 w154 w242] -> w48
      tunnel: [w60 w153 w241] -> w47
      frame "Camera On" {
        n11 = call <vilib>:"IMAQdx Grab2.vi"("Image In"=w68, "Session In"=w69) -> ("Image Out"=w57:T11, "Session Out"=w66:T13)  [unwired: 6 in, 2 out]
        "Color" <- w57
        n12 = case shown="True" "Color Sampling" {
          tunnel: w65 -> [w89 w122]
          tunnel: w64 -> [w90 w121]
          tunnel: w63 -> [w92 w120]
          tunnel: w57 -> [w105 w118]
          tunnel: "Color Index" -> [w109 w119]
          tunnel: [w73 w122] -> w61
          tunnel: [w72 w121] -> w60
          tunnel: [w74 w120] -> w59
          tunnel: [w75 w118] -> w58
          frame False {
            w77 = T10[] [enum."R", enum."G", enum."B", enum."Y", enum."K"] items=["R", "G", "B", "Y", "K"]
            w93 = u16 2 items=["RGB", "HSL", "HSV", "HSI"] ("Color Mode")
            w94 = u16 2 items=["RGB", "HSL", "HSV", "HSI"] ("Color Mode")
            w95 = u16 2 items=["RGB", "HSL", "HSV", "HSI"] ("Color Mode")
            n13 = property on="Color" class="ImageControl"() -> ("ROI"=w116:T14)  [unwired: 2 in, 2 out]
            n14 = Unbundle By Name(w116) -> ("Global Rectangle"=w115:i32[])
            n15 = Index Array(array="HSV Sample", index #1=w109, index #2=1 ("index"), index #3=2 ("index")) -> (element #1=w108:T15, element #2=w107:T15, element #3=w106:T15)
            n16 = call "IMAQ Extract 2"("Y Step Size"=0, "Optional Rectangle"=w115, "X Step Size"=0, "Image Src"=w105) -> ("Image Dst Out"=w91:T11)  [unwired: 6 in, 1 out]
            n17 = Unbundle By Name(w108) -> ("Red or Hue Range"=w98:cluster{"Lower value":i32, "Upper value":i32}, "Green or Sat Range"=w97:cluster{"Lower value":i32, "Upper value":i32}, "Blue or Luma or Val or Inten Range"=w96:cluster{"Lower value":i32, "Upper value":i32})
            n18 = Unbundle By Name(w107) -> ("Red or Hue Range"=w104:cluster{"Lower value":i32, "Upper value":i32}, "Green or Sat Range"=w103:cluster{"Lower value":i32, "Upper value":i32}, "Blue or Luma or Val or Inten Range"=w102:cluster{"Lower value":i32, "Upper value":i32})
            n19 = Unbundle By Name(w106) -> ("Red or Hue Range"=w101:cluster{"Lower value":i32, "Upper value":i32}, "Green or Sat Range"=w100:cluster{"Lower value":i32, "Upper value":i32}, "Blue or Luma or Val or Inten Range"=w99:cluster{"Lower value":i32, "Upper value":i32})
            n20 = call "IMAQ ColorThreshold"("Blue or Luma or Val or Inten Range"=w96, "Green or Sat Range"=w97, "Color Mode"=w95, "Red or Hue Range"=w98, "Image Dst"=w92, "Image Src"=w91) -> ("Image Dst Out"=w72:T11)  [unwired: 4 in, 1 out]
            "Particle" <- w72
            n21 = call "IMAQ ColorThreshold"("Blue or Luma or Val or Inten Range"=w102, "Green or Sat Range"=w103, "Color Mode"=w94, "Red or Hue Range"=w104, "Image Dst"=w90, "Image Src"=w91) -> ("Image Dst Out"=w71:T11)  [unwired: 4 in, 1 out]
            "Particle 2" <- w71
            n22 = call "IMAQ ColorThreshold"("Blue or Luma or Val or Inten Range"=w99, "Green or Sat Range"=w100, "Color Mode"=w93, "Red or Hue Range"=w101, "Image Dst"=w89, "Image Src"=w91) -> ("Image Dst Out"=w70:T11)  [unwired: 4 in, 1 out]
            "Particle 3" <- w70
            n23 = call "IMAQ Particle Analysis Report"("Image"=w72) -> ("Particle Reports (Pixels)"=w88:T16, "Image Out (duplicate)"=w75:T11)  [unwired: 5 in, 4 out]
            n24 = call "IMAQ Particle Analysis Report"("Image"=w71) -> ("Particle Reports (Pixels)"=w87:T16, "Image Out (duplicate)"=w74:T11)  [unwired: 5 in, 4 out]
            n25 = call "IMAQ Particle Analysis Report"("Image"=w70) -> ("Particle Reports (Pixels)"=w86:T16, "Image Out (duplicate)"=w73:T11)  [unwired: 5 in, 4 out]
            n26 = Array Max & Min(array=w86) -> (max value=w83:T17)  [unwired: 3 out]
            n27 = Array Max & Min(array=w87) -> (max value=w84:T17)  [unwired: 3 out]
            n28 = Array Max & Min(array=w88) -> (max value=w85:T17)  [unwired: 3 out]
            n29 = Unbundle By Name(w85) -> ("Area"=w81:dbl)
            n30 = Unbundle By Name(w84) -> ("Area"=w82:dbl)
            n31 = Unbundle By Name(w83) -> ("Area"=w80:dbl)
            n32 = Build Array(w81, w82, w80) -> (w79:dbl[])
            n33 = Array Max & Min(array=w79) -> (max index (indices)=w78:i32)  [unwired: 3 out]
            n34 = Index Array(array=w77, index=w78) -> (element=→"color element":T10)
          }
          frame True {
            w125 = u16 2 items=["RGB", "HSL", "HSV", "HSI", "CIE L*a*b*", "CIE XYZ"] ("Color Mode")
            n35 = property on="Color" class="ImageControl"() -> ("ROI"=w148:T14)  [unwired: 2 in, 2 out]
            n36 = Unbundle By Name(w148) -> ("Global Rectangle"=w147:i32[])
            n37 = call "IMAQ Extract 2"("Y Step Size"=0, "Optional Rectangle"=w147, "X Step Size"=0, "Image Src"=w118) -> ("Image Dst Out"=w117:T11)  [unwired: 6 in, 1 out]
            "ROI" <- w117
            n38 = call "IMAQ ColorHistogram"("Color Mode"=w125, "Image Src"=w117) -> ("Red or Hue or X or L* Histogram Report"=w144:T18, "Green or Sat or Y or a* Histogram Report"=w143:T18, "Blue or Luma or Val or Inten or Z or b* Histogram Report"=w142:T18)  [unwired: 4 in, 1 out]
            n39 = Unbundle By Name(w144) -> ("Minimal Value"=w141:sgl, "Maximal Value"=w140:sgl)
            n40 = Unbundle By Name(w143) -> ("Minimal Value"=w139:sgl, "Maximal Value"=w138:sgl)
            n41 = Unbundle By Name(w142) -> ("Minimal Value"=w137:sgl, "Maximal Value"=w136:sgl)
            n42 = To Long Integer(number=w141) -> (32bit integer=w135:i32)
            n43 = To Long Integer(number=w140) -> (32bit integer=w134:i32)
            n44 = To Long Integer(number=w137) -> (32bit integer=w131:i32)
            n45 = To Long Integer(number=w136) -> (32bit integer=w130:i32)
            n46 = To Long Integer(number=w139) -> (32bit integer=w133:i32)
            n47 = To Long Integer(number=w138) -> (32bit integer=w132:i32)
            n48 = Bundle(w133, w132) -> (w128:cluster{i32, i32})  [unwired: 1 in]
            n49 = Bundle(w135, w134) -> (w129:cluster{i32, i32})  [unwired: 1 in]
            n50 = Bundle(w131, w130) -> (w127:cluster{i32, i32})  [unwired: 1 in]
            n51 = local read "HSV Sample"() -> (w123:T12)
            n52 = Bundle(w129, w128, w127) -> (w126:T19)  [unwired: 1 in]
            n53 = Insert Into Array(array=w123, index=w119, new element=w126) -> (w124:T12)
            n54 = local write "HSV Sample"(w124) -> ()
          }
        }
      }
      frame "Scan QR" {
        w165 = 1 items=["Red", "Green", "Blue", "Hue", "Saturation", "Luminance", "Value", "Intensity"] ("Color Plane")
        n55 = call <vilib>:"IMAQdx Grab2.vi"("Image In"=w170, "Session In"=w169) -> ("Image Out"=w153:T11, "Session Out"=w154:T13)  [unwired: 6 in, 2 out]
        n56 = call "IMAQ ExtractSingleColorPlane"("Color Plane"=w165, "Image Src"=w153) -> ("Image Dst Out"=w168:T11)  [unwired: 8 in, 1 out]
        n57 = call "IMAQ Read QR Code"("QR Code Cell Size (pixels)"="QR Code Cell Size (pixels)", "QR Search Options"="QR Search Options", "QR Description Options"="QR Description Options", "Image"=w168) -> ("QR Code Report"=w163:T20, "Image (duplicate)"=→"Image":T11)  [unwired: 4 in, 2 out]
        n58 = local read "Data num"() -> (w160:dbl)
        n59 = Unbundle By Name(w163) -> ("Found?"=w162:bool, "Data"=w161:string)
        "Found?" <- w162
        "Data" <- w161
        n60 = To Long Integer(number=w160) -> (32bit integer=w159:i32)
        n61 = case shown="True" w162 {
          tunnel: w161 -> [_ w214]
          tunnel: w159 -> [_ w173]
          tunnel: [w171 w172] -> w158
          frame False {
            n62 = local read "output cluster"() -> (w171:cluster{"Kota":T9, T10[], bool[]})
          }
          frame True {
            n63 = String Subset(string=w214, offset (0)=1, length (rest)=1 ("length (rest)")) -> (substring=w230:string)
            n64 = String Subset(string=w214, offset (0)=2, length (rest)=1 ("length (rest)")) -> (substring=w227:string)
            n65 = String Subset(string=w214, offset (0)=3, length (rest)=1 ("length (rest)")) -> (substring=w224:string)
            n66 = String Subset(string=w214, offset (0)=4, length (rest)=1 ("length (rest)")) -> (substring=w217:string)
            n67 = String Subset(string=w214, offset (0)=5, length (rest)=1 ("length (rest)")) -> (substring=w216:string)
            n68 = String Subset(string=w214, offset (0)=6, length (rest)=1 ("length (rest)")) -> (substring=w215:string)
            n69 = Equal?(x=w217, y="1" ("Item 2")) -> (x = y?=w199:bool)
            n70 = Equal?(x=w216, y="1" ("Item 2")) -> (x = y?=w198:bool)
            n71 = Equal?(x=w215, y="1" ("Item 2")) -> (x = y?=w197:bool)
            n72 = Scan From String(input string=w230, default 1=Barang."R") -> (error out=w210:errorcluster, output 1=w202:T10)  [unwired: 3 in, 2 out]
            n73 = Scan From String(input string=w224, default 1=Barang."B") -> (error out=w208:errorcluster, output 1=w200:T10)  [unwired: 3 in, 2 out]
            n74 = Scan From String(input string=w227, default 1=Barang."G") -> (error out=w209:errorcluster, output 1=w201:T10)  [unwired: 3 in, 2 out]
            n75 = String Subset(string=w214, offset (0)=0, length (rest)=1 ("length (rest)")) -> (substring=w212:string)
            n76 = Scan From String(input string=w212, default 1=Kota."Unidentified" ("Kota")) -> (error out=w211:errorcluster, output 1=w184:T9)  [unwired: 3 in, 2 out]
            n77 = Merge Errors(w211, w210, w209, w208) -> (w207:errorcluster)
            n78 = Bundle(w202, w199) -> (w203:cluster{T10, bool})  [unwired: 1 in]
            n79 = Bundle(w201, w198) -> (w204:cluster{T10, bool})  [unwired: 1 in]
            n80 = Bundle(w200, w197) -> (w205:cluster{T10, bool})  [unwired: 1 in]
            n81 = Unbundle By Name(w207) -> ()  [unwired: 1 out]
            n82 = Build Array(w203, w204, w205) -> (w206:cluster{T10, bool}[])
            n83 = Sort 1D Array(array=w206) -> (sorted array=w189:cluster{T10, bool}[])
            n84 = Index Array(array=w189, index #2=0 ("index")) -> (element #1=w196:cluster{T10, bool}, element #2=w188:cluster{T10, bool}, element #3=w187:cluster{T10, bool})  [unwired: 2 in]
            n85 = Unbundle(w196) -> (w195:T10, w192:bool)
            n86 = Unbundle(w188) -> (w194:T10, w191:bool)
            n87 = Unbundle(w187) -> (w193:T10, w190:bool)
            n88 = Build Array(w195, w194, w193) -> (w186:T10[])
            n89 = Build Array(w192, w191, w190) -> (w185:bool[])
            n90 = Bundle("Kota"=w184, w186, w185) -> (w172:cluster{"Kota":T9, T10[], bool[]})  [unwired: 1 in]
            "output cluster" <- w172
            n91 = feedback #1(cluster{"Kota":T9, T10[], bool[]}[] [{"Kota"=enum."Unidentified", [], []}, {"Kota"=enum."Unidentified", [], []}, {"Kota"=enum."Unidentified", [], []}, {"Kota"=enum."Unidentified", [], []}]) -> (w183:cluster{"Kota":T9, T10[], bool[]}[])
            n92 = Replace Array Subset(array=w183, new element=w172, index=w173) -> (w181:cluster{"Kota":T9, T10[], bool[]}[])
            n93 = feedback-in #1(w181) -> ()
            n94 = Index Array(array=w181, index #1=0 ("index")) -> (element #1=w179:cluster{"Kota":T9, T10[], bool[]}, element #2=w178:cluster{"Kota":T9, T10[], bool[]}, element #3=w177:cluster{"Kota":T9, T10[], bool[]}, element #4=w176:cluster{"Kota":T9, T10[], bool[]})  [unwired: 3 in]
            n95 = Build Array(w178, w179, w176, w177) -> (→"appended array":cluster{"Kota":T9, T10[], bool[]}[])
          }
        }
        n96 = Unbundle By Name(w158) -> ("Kota"=w156:T9)
        n97 = Not Equal?(x=w156, y=Kota."Unidentified" ("Kota")) -> (x != y?=→"Saved":bool)
      }
      frame "Camera Off", Default {
      }
    }
    n98 = Unbundle By Name(w42) -> ("X axis"=w27:i32, "Y axis"=w26:i32, "Z axis"=w25:i32)
    n99 = Wait (ms)(milliseconds to wait=u32 1) -> ()  [unwired: 1 out]
    n100 = Divide(x=w27, y=-32768) -> (x/y=w31:dbl)
    n101 = Divide(x=w26, y=32768) -> (x/y=w33:dbl)
    n102 = Divide(x=w25, y=-32768) -> (x/y=w35:dbl)
    n103 = Multiply(x=w31, y=250.0) -> (x*y=w37:dbl)
    n104 = Multiply(x=w33, y=250.0) -> (x*y=w38:dbl)
    n105 = Multiply(x=w35, y=10.0) -> (x*y=w39:dbl)
    n106 = Build Array(w37, w38, w39) -> (w40:dbl[])
    n107 = shared-variable "My Computer\\test.lvlib\\Variable3"(w40) -> ()  [unwired: 1 in, 1 out]
  }
  n108 = call-poly <vilib>:"Close Input Device.vi"("error in (no error)"=w1, "device ID"=w3) -> ("error out"=→"error out":errorcluster)  [unwired: 8 in]
  n109 = call "IMAQ Dispose"("Image"=w9) -> ()  [unwired: 5 in, 1 out]
  n110 = call "IMAQ Dispose"("Image"=w8) -> ()  [unwired: 5 in, 1 out]
  n111 = call <vilib>:"IMAQdx Close Camera.vi"("Session In"=w10) -> ()  [unwired: 10 in, 1 out]
  n112 = call "IMAQ Dispose"("Image"=w6) -> ()  [unwired: 5 in, 1 out]
  n113 = call "IMAQ Dispose"("Image"=w7) -> ()  [unwired: 5 in, 1 out]
